vi "main mapping.vi"(8 "error in":errorcluster) -> (0 "error out":errorcluster)   [LabVIEW 2023]
uses:
  control/Data Form.ctl
  control/rois list cluster.ctl
  control/param_calibrazione.ctl
  <vilib>/Utility/miscctls.llb/LVStringsAndValuesArrayTypeDef_I16.ctl
  <vilib>/Utility/file.llb/Write Delimited Spreadsheet (I64).vi
  <vilib>/Utility/file.llb/Read Delimited Spreadsheet (string).vi
  queue/Front Panel Message Queue.lvlib
panel:
  in  "crop Z":bool
  in  "Crop Z sl":cluster{i32, i32}(slide) scale=0.0..10.0
  out "Invert Roi XY":bool[](array[boolean])
  out "Roi XY":T1
  in  "crop all":bool
  in  "crop":bool
  in  "save all":bool
  in  "save":bool
  in  "export":bool
  in  "Edit ROI":bool
  in  "autoscale":bool
  out "Calibration":T2
  in  "manipulate files":bool
  in  "area ROI":bool
  out "ROIs Values":string[][](table)
  out "data ROIs":T3
  out "ROIs Values Data":dbl[][](array[numeric])
  in  "ROIs List":i16(ring) items=["All", "Ca - Escape Peak", "S - Ka1", "Cl - Ka1", "Ar - Ka1", "K - Ka1", "Ca - Ka1", "Ca - Kb1", "Ti - Ka1", "Mn - Ka1", "Fe - Ka1", "Fe - Kb1", "Cu - Ka1", "Zn - Ka1"]
  in  "debug?":bool
  in  "load param":bool
  in  "load calib":bool
  in  "calibrate":bool
  in  "mapping":enum16{"Y - Linear", "Y - Log"}(ring)
  out "Intensity Graph":i32[][](graph)
  in  "reset":bool
  in  "reset ROI":bool
  out "Sum Spectrum":cluster{"Ramp Pattern":dbl[], "Array":i32[]}[](graph)
  in  "load data":bool
  in  "Data Form":T4={"Dimensions"={"Dim X"=0, "Dim Y"=0, "Dim Z"=0}, "Folder XRF Files"=path "", "Dynamic Load"=FALSE, "Data From Vitruvio?"=TRUE}
  in  "Z Slice":i16(slide) scale=0.0..10.0
  in  "Stop":bool
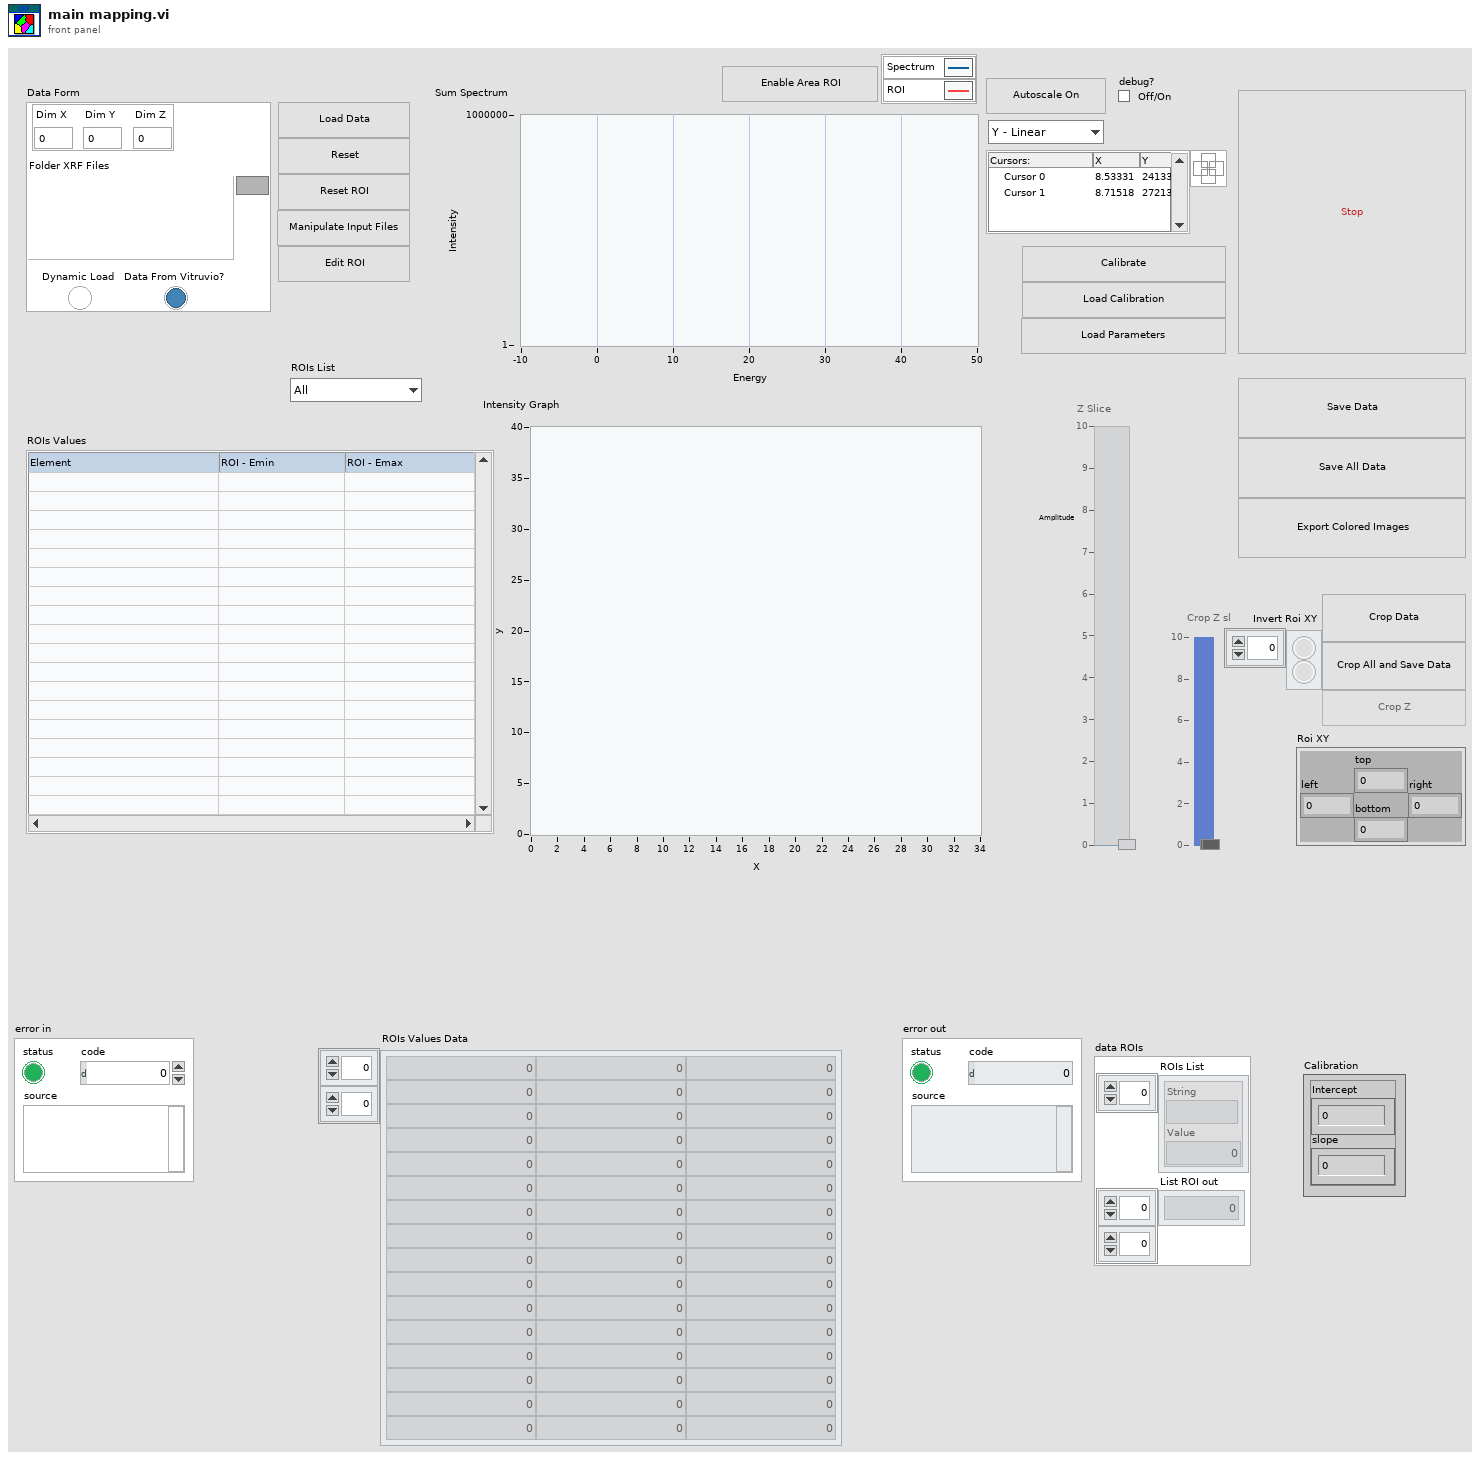
[diagram p1: front panel]
types:
  T1 = cluster{"left":i16, "top":i16, "right":i16, "bottom":i16}
  T2 = typedef "param_calibrazione.ctl" = cluster{"Intercept":dbl, "slope":dbl}
  T3 = typedef "rois list cluster.ctl" = cluster{"ROIs List":cluster{"String":string, "Value":i32}[], "List ROI out":dbl[][]}
  T4 = typedef "Data Form.ctl" = cluster{"Dimensions":cluster{"Dim X":i32, "Dim Y":i32, "Dim Z":i32}, "Folder XRF Files":path, "Dynamic Load":bool, "Data From Vitruvio?":bool}
  T5 = enum8{"Enabled", "Disabled", "Disabled and Grayed Out"}
  T6 = typedef "Front Panel Message Queue.lvlib/load 3 Messages Queues.ctl" = cluster{"Main":refnum<queue>, "Data":refnum<queue>, "Support":refnum<queue>}
  T7 = typedef "LVStringsAndValuesArrayTypeDef_I16.ctl" = cluster{"String":string, "Value":i16}[]
  T8 = typedef "LVRowAndColumnTypeDef.ctl" = cluster{"Row":i32, "Column":i32}
  T9 = typedef "LVCursorListTypeDef.ctl" = cluster{"Name":string, "Color":u32, "Style":u8, "Point Style":u8, "Name Visible":bool, "Allow Drag":bool, "Cursor Mode":u32, "Plot":i32, "Index":i32, "Position":cluster{"X":dbl, "Y":dbl}, "X Scale":u32, "Y Scale":u32, "Watch Plots":i32[], "Watch All Plots":bool, "Plot Area":i32, "Label Offset":cluster{"X":dbl, "Y":dbl}}[]
  T10 = cluster{"Name":string, "Color":u32, "Style":u8, "Point Style":u8, "Name Visible":bool, "Allow Drag":bool, "Cursor Mode":u32, "Plot":i32, "Index":i32, "Position":cluster{"X":dbl, "Y":dbl}, "X Scale":u32, "Y Scale":u32, "Watch Plots":i32[], "Watch All Plots":bool, "Plot Area":i32, "Label Offset":cluster{"X":dbl, "Y":dbl}}
  T11 = cluster{"Name":string, "Color":u32, "Style":u8, "Point Style":u8, "Name Visible":bool, "Allow Drag":bool, "Cursor Mode":u32, "Plot":i32, "Index":i32, "Position":cluster{"X":dbl, "Y":dbl}, "X Scale":u32, "Y Scale":u32, "Watch Plots":i32[], "Watch All Plots":bool, "Plot Area":i32, "Label Offset":cluster{"X":dbl, "Y":dbl}}[]
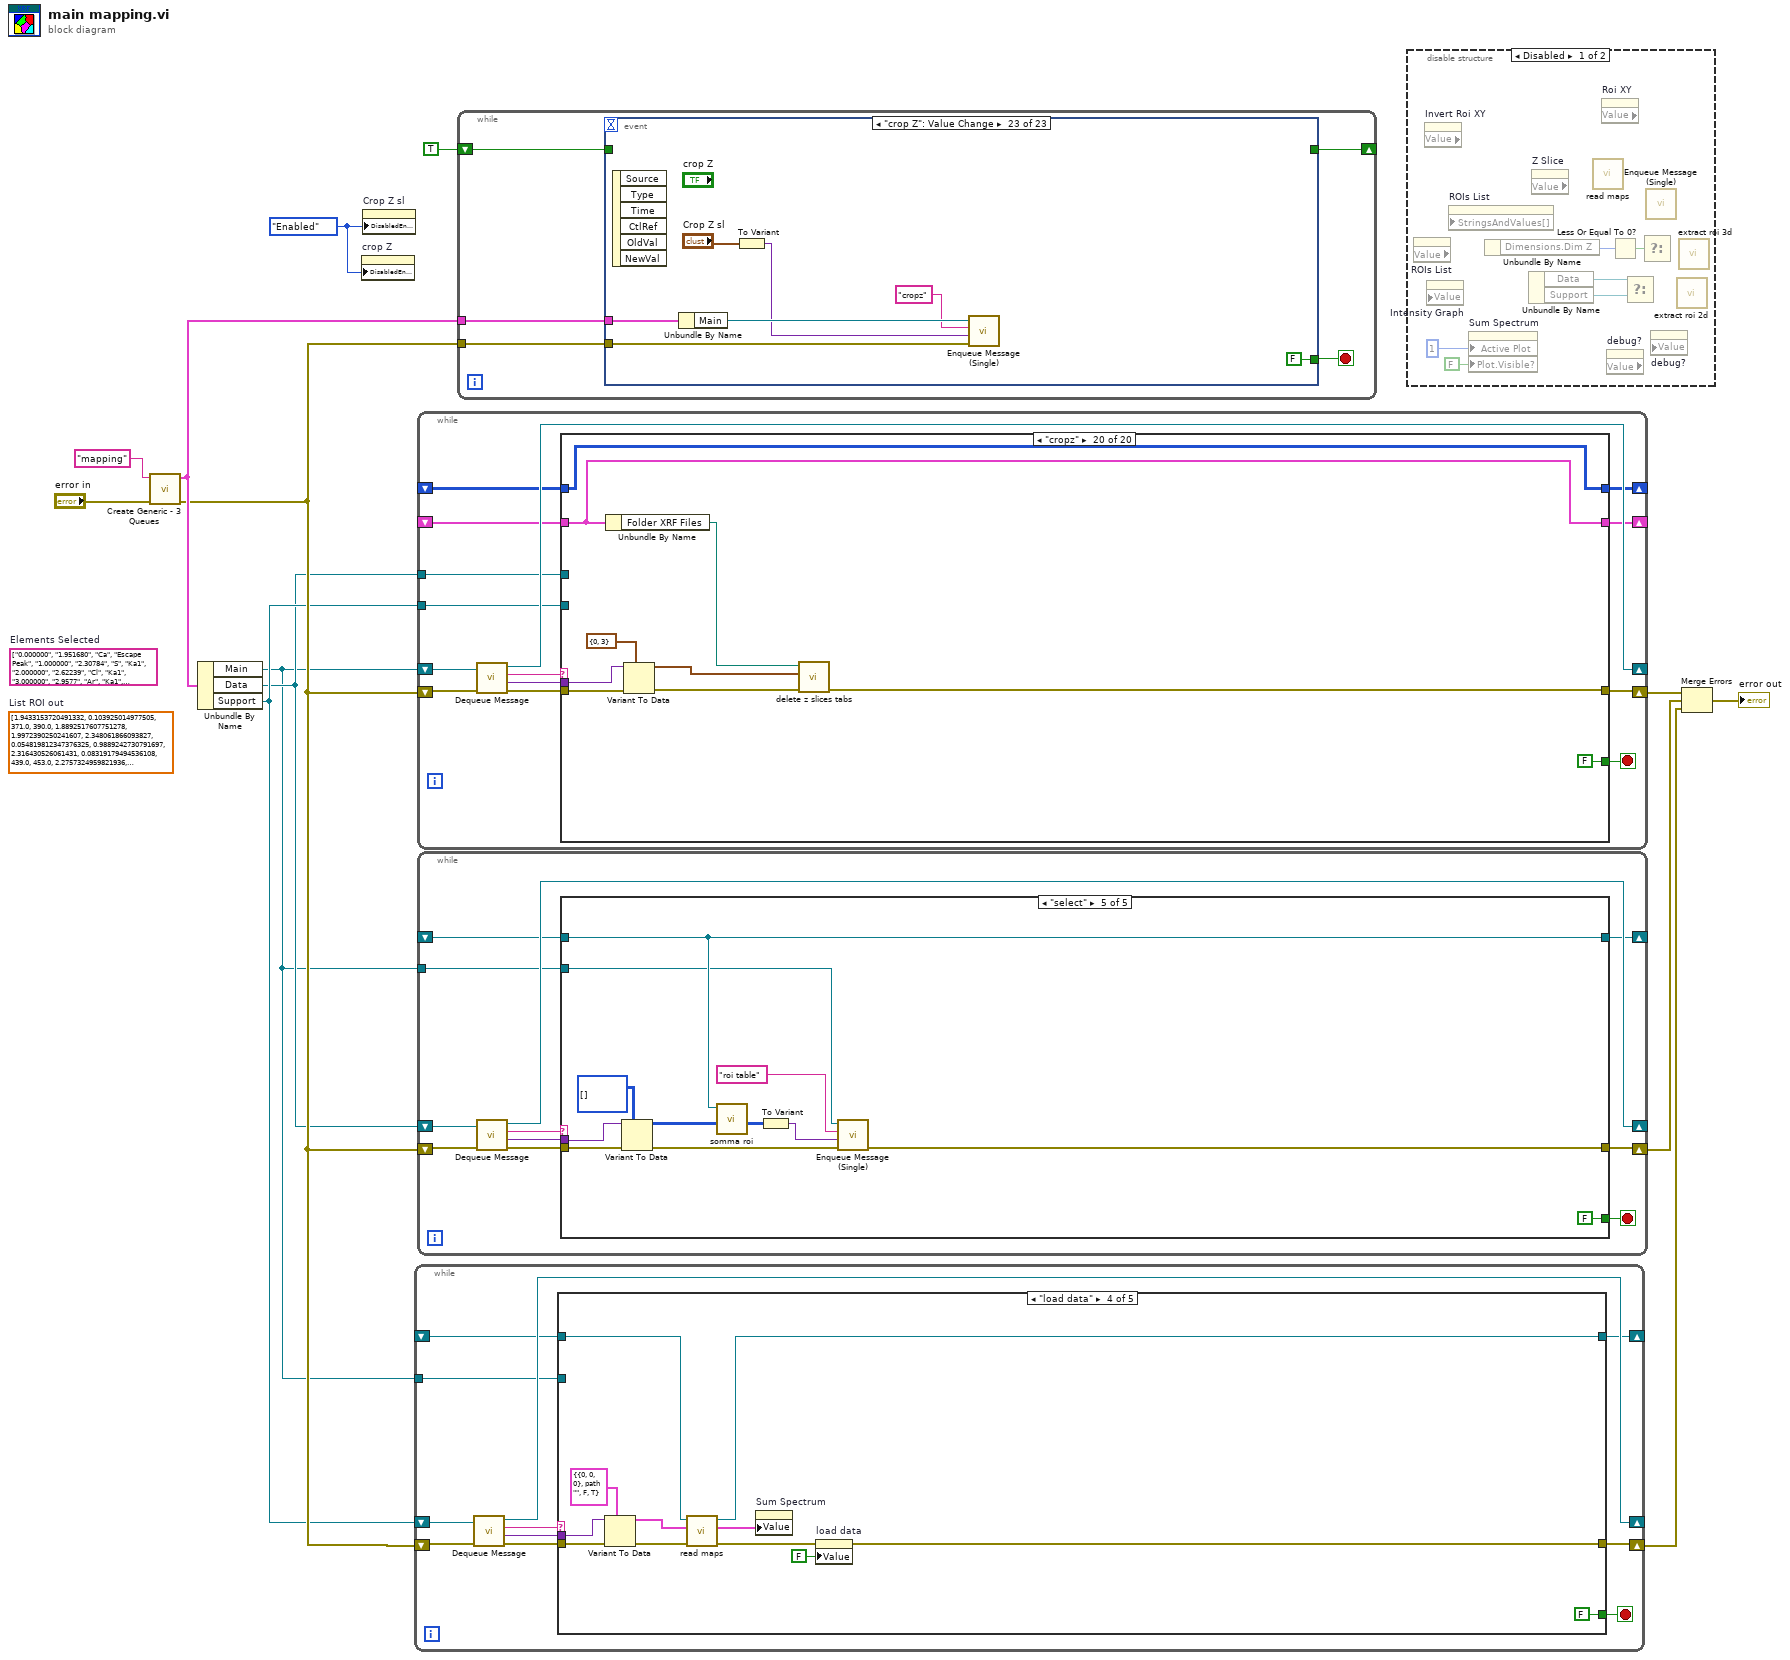
[diagram p0: block diagram]
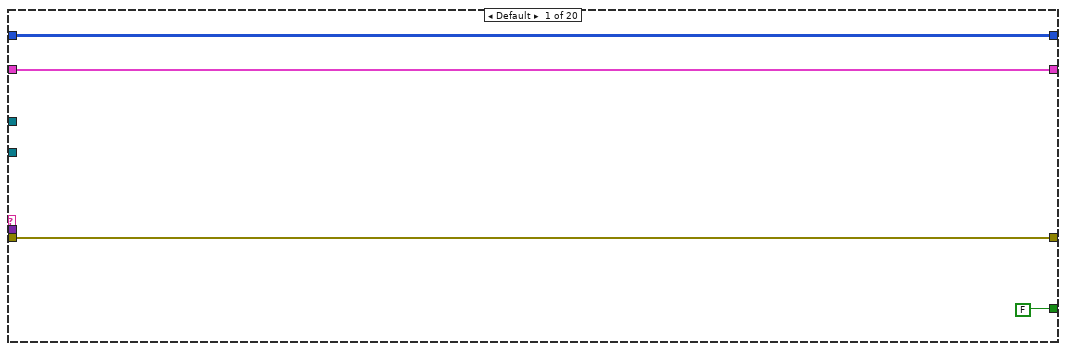
[diagram p3: hidden frame]
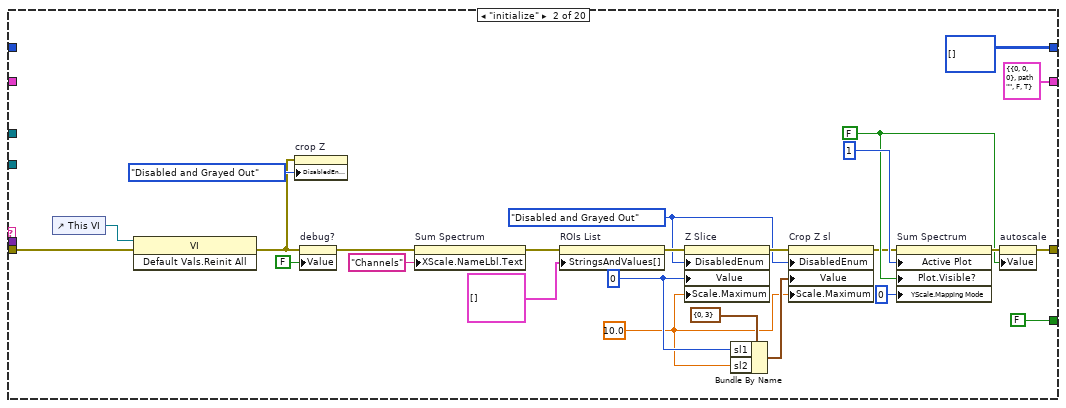
[diagram p4: hidden frame]
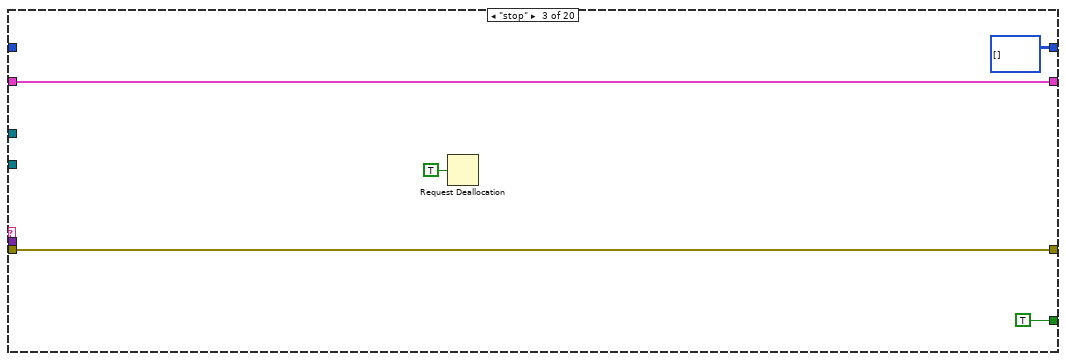
[diagram p5: hidden frame]
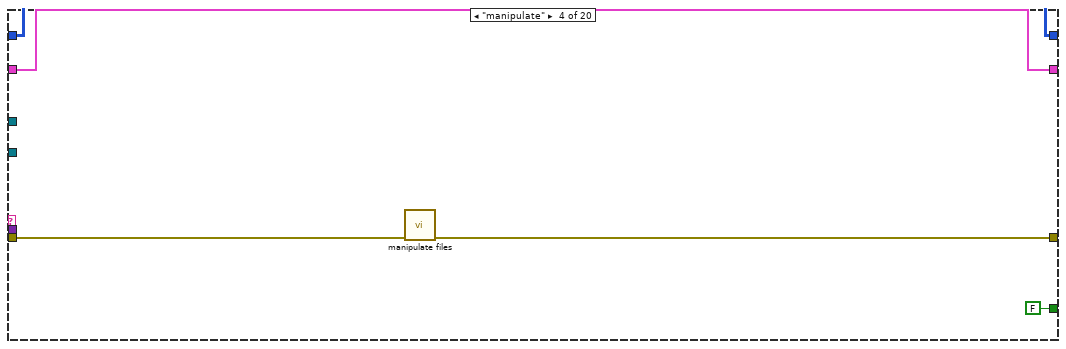
[diagram p6: hidden frame]
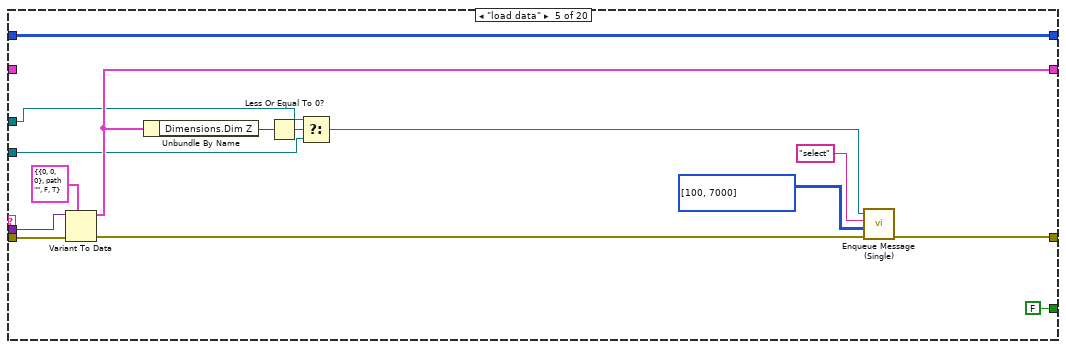
[diagram p7: hidden frame]
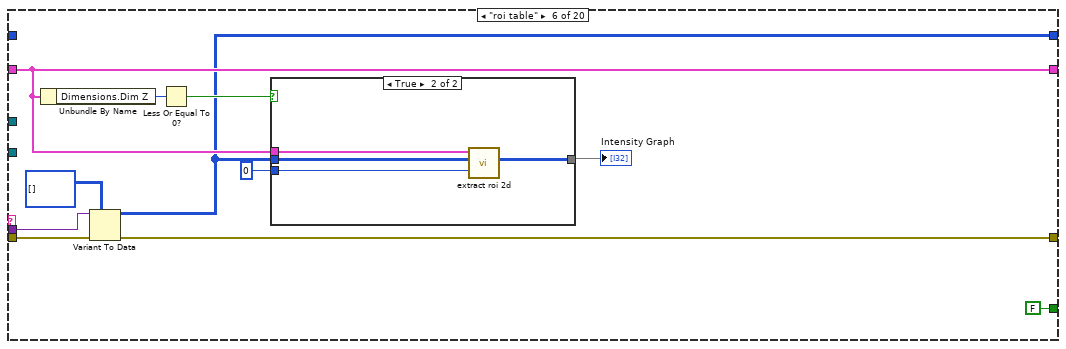
[diagram p8: hidden frame]
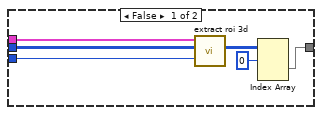
[diagram p9: hidden frame]
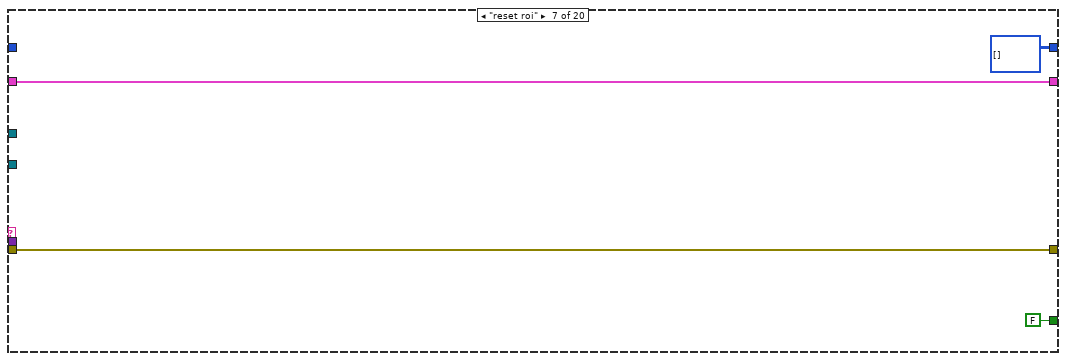
[diagram p10: hidden frame]
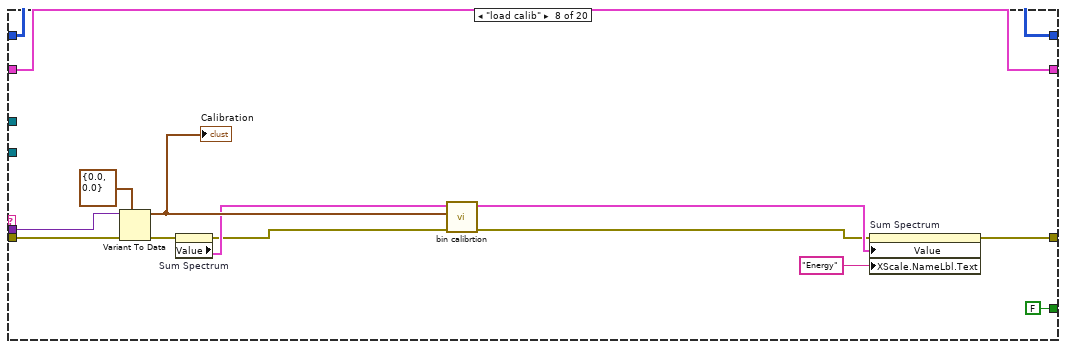
[diagram p11: hidden frame]
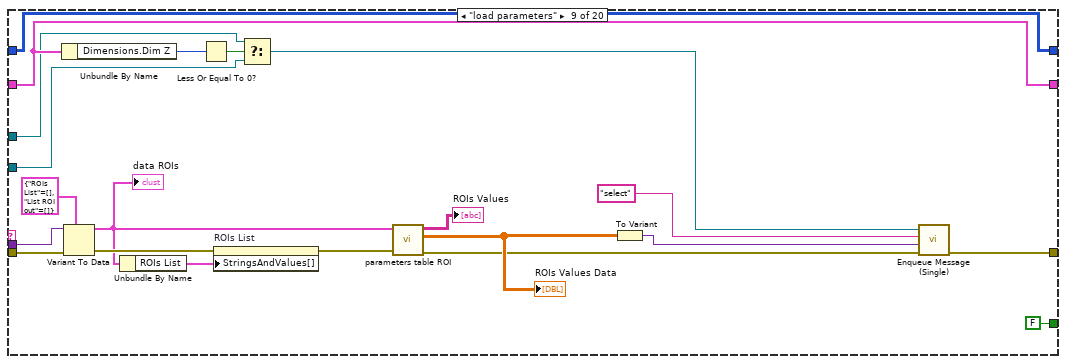
[diagram p12: hidden frame]
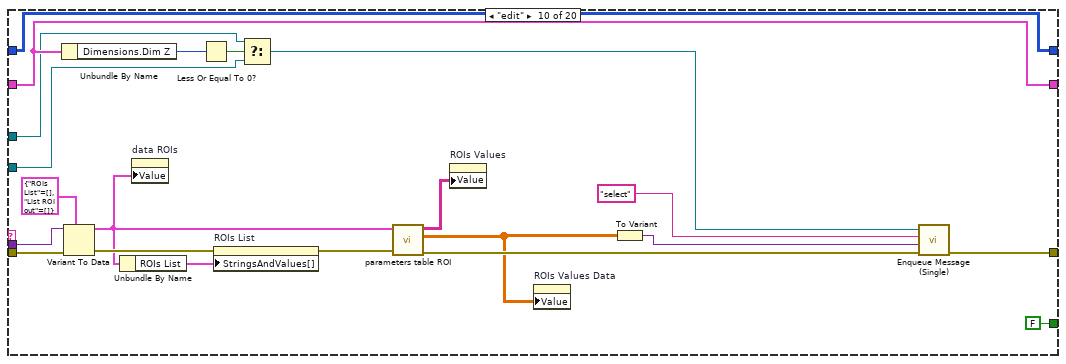
[diagram p13: hidden frame]
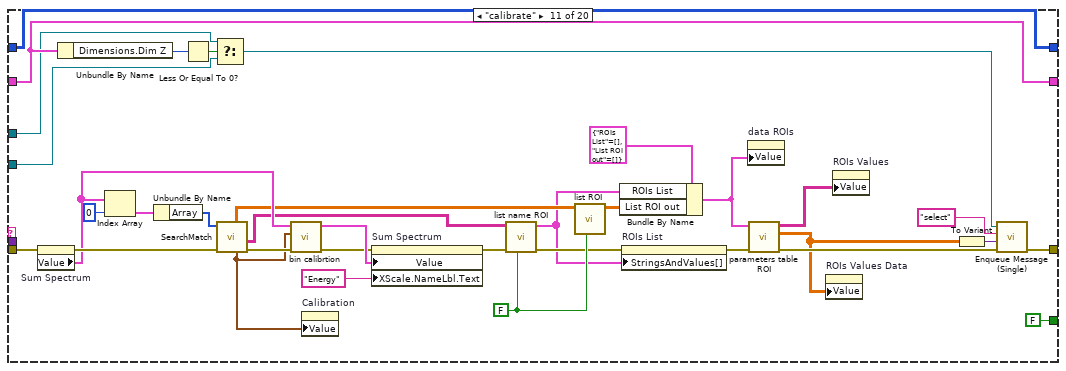
[diagram p14: hidden frame]
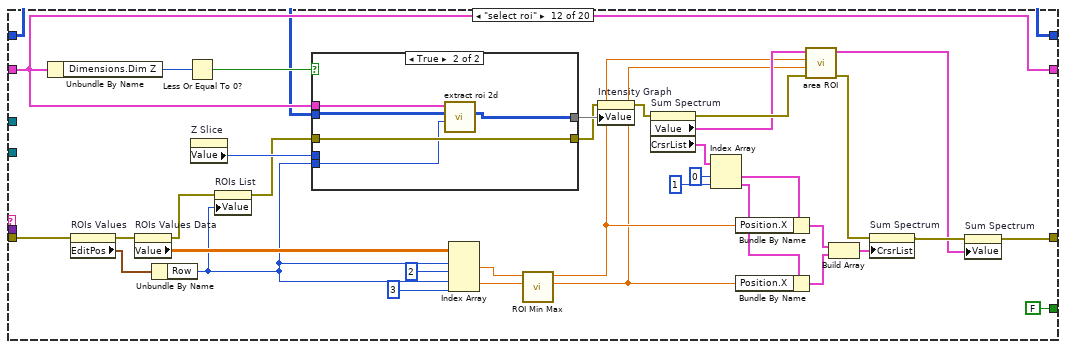
[diagram p15: hidden frame]
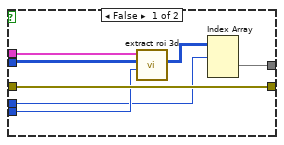
[diagram p16: hidden frame]
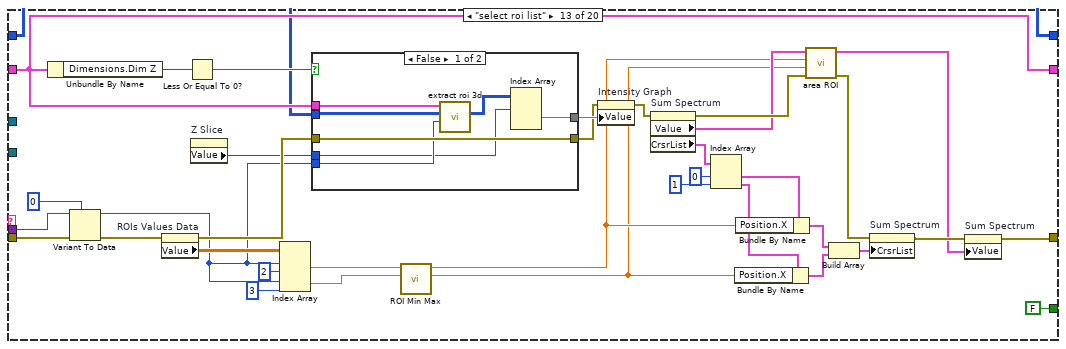
[diagram p17: hidden frame]
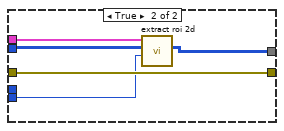
[diagram p18: hidden frame]
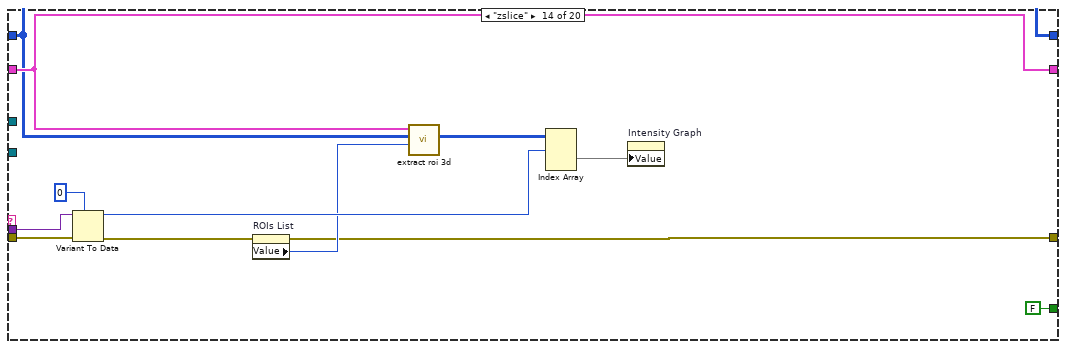
[diagram p19: hidden frame]
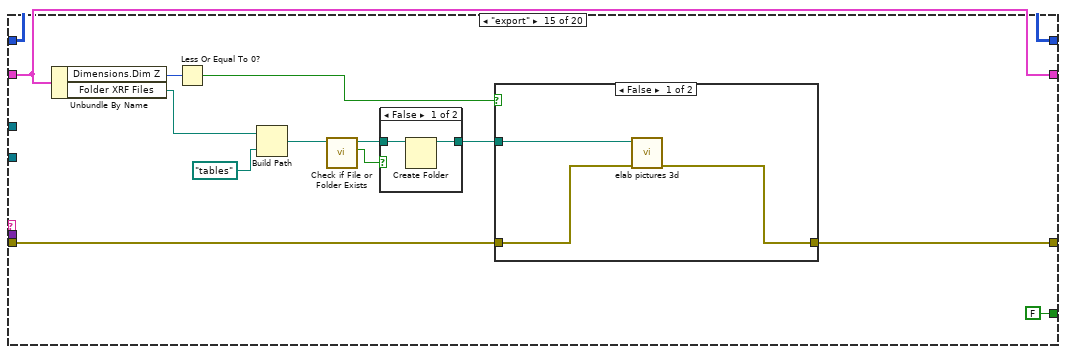
[diagram p20: hidden frame]
diagram:
  w1 = T5."Enabled" ("Disabled")
  (unwired) string[][] [["0.000000", "1.951680", "Ca", "Escape Peak"], ["1.000000", "2.30784", "S", "Ka1"], ["2.000000", "2.62239", "Cl", "Ka1"], ["3.000000", "2.9577", "Ar", "Ka1"], ["4.000000", "3.3138", "K", "Ka1"], ["5.000000", "3.69168", "Ca", "Ka1"], ["6.000000", "4.0127", "Ca", "Kb1"], ["7.000000", "4.51084", "Ti", "Ka1"], ["8.000000", "5.89875", "Mn", "Ka1"], ["9.000000", "6.40384", "Fe", "Ka1"], ["10.000000", "7.05798", "Fe", "Kb1"], ["11.000000", "8.04778", "Cu", "Ka1"], ["12.000000", "8.63886", "Zn", "Ka1"]]  # Elements Selected
  (unwired) dbl[][] [[1.9433153720491332, 0.103925014977505, 371.0, 390.0, 1.8892517607751278, 1.9972390250241607, 2.348061866093827, 0.054819812347376325, 0.9889242730791697], [2.316430526061431, 0.08319179494536108, 439.0, 453.0, 2.2757324959821936, 2.3553020591130602, 1.2026044683685715, 0.06508434345467039, 0.9422897397723133], [2.6291250873578926, 0.09464714383641912, 493.0, 510.0, 2.5826436680583935, 2.67926385186016, 6.041240478814808, 0.09369315412168325, 0.9948773271231875], [2.9638857471497273, 0.10205305258568396, 551.0, 569.0, 2.912289001029126, 3.0145927250545257, 19.912809301577955, 0.16530990532407933, 0.9985039668315457], [3.315602816840393, 0.10433962779562063, 613.0, 631.0, 3.264668494894392, 3.366972218919792, 7.760413909880946, 0.3328586753679668, 0.960961680843631], [3.695302221205313, 0.11473980336266298, 679.0, 699.0, 3.6397821496541916, 3.7534529541268578, 209.52164584521063, 0.9542698579126939, 0.9995310820008576], [4.016866195819118, 0.11712275853598021, 735.0, 756.0, 3.9580604021776575, 4.0774147468739566, 31.75496431275371, 0.47134819167031033, 0.9949696927449659], [4.512431596555036, 0.12331628047684387, 822.0, 843.0, 4.4525284016337565, 4.571882746330056, 2.030401395630214, 0.06554154967612931, 0.9764849440574406], [5.899492088990847, 0.14789502732767537, 1064.0, 1090.0, 5.827945135753021, 5.975717181567487, 2.129686188635054, 0.14744421626074894, 0.8984068833785415], [6.3992920200960155, 0.14207300042877877, 1152.0, 1177.0, 6.328096675432753, 6.470185181023586, 53.24985306608518, 0.5108773919278868, 0.9977288374603356], [7.060693940644275, 0.1502701906643122, 1268.0, 1294.0, 6.987387341374219, 7.135159387188685, 7.411818206694545, 0.3851918524072267, 0.9365265800601416], [8.037279832035043, 0.15266067897053234, 1439.0, 1466.0, 7.959272719615518, 8.112728305653617, 8.778131477093314, 0.519491476790709, 0.9143052423937907], [8.624129113105631, 0.1800441786593039, 1540.0, 1572.0, 8.533310282202482, 8.715183569358748, 10.127705234792012, 0.49635854961799064, 0.9435596103561451]]  # List ROI out
  n1 = call "Create Generic - 3 Queues.vi"("error in (no error)"="error in", "name"="mapping") -> ("error out"=w7:errorcluster, "Message Queues"=w11:T6)  [unwired: 8 in]
  n2 = Unbundle By Name(w11) -> ("Main"=w2:refnum<queue>, "Data"=w5:refnum<queue>, "Support"=w6:refnum<queue>)
  n3 = property on="crop Z" class="Bool"("DisabledEnum"=w1) -> ()  [unwired: 2 in, 2 out]
  n4 = property on="Crop Z sl" class="Slide (strict)"("DisabledEnum"=w1) -> ()  [unwired: 2 in, 2 out]
  n5 = while {
    shift-right: [w22] -> _
    shift-left: w6 -> [w23]
    shift-right: [w17] -> w9
    shift-left: w7 -> [w24]
    shift-right: [w16] -> _
    shift-left: _ -> [w15]
    tunnel: w2 -> [w14]
    stop <- w19 stop-if-true
    n6 = call "Dequeue Message.vi"("error in (no error)"=w24, "Message Queue"=w23) -> ("error out"=w21:errorcluster, "Message Data"=w18:variant, "Message"=w20:string, "dup Message Queue"=w22:refnum<queue>)  [unwired: 5 in, 1 out]
    n7 = case shown="\"load data\"" w20 {
      tunnel: w21 -> [w26 w28 w36 w47 w58]
      tunnel: [FALSE FALSE TRUE FALSE FALSE] -> w19
      tunnel: w18 -> [_ _ _ w46 w59]
      tunnel: [w26 w29 w35 w38 w50] -> w17
      tunnel: [w25 w30 refnum<data-value> refnum ("data value reference out") w41 w57] -> w16
      tunnel: w15 -> [w25 _ w34 w44 w57]
      tunnel: w14 -> [_ _ _ _ w51]
      frame Default {
      }
      frame "initialize" {
        n8 = New Data Value Reference(data value=i32[][] [] ("Data Loaded"), error in=w28) -> (data value reference=w30:refnum<data-value>, error out=w29:errorcluster)
      }
      frame "stop" {
        n9 = Delete Data Value Reference(data value reference=w34, error in=w36) -> (error out=w35:errorcluster)  [unwired: 1 out]
      }
      frame "load data" {
        n10 = Variant To Data(error in=w47, type=T4 {"Dimensions"={"Dim X"=0, "Dim Y"=0, "Dim Z"=0}, "Folder XRF Files"=path "", "Dynamic Load"=FALSE, "Data From Vitruvio?"=TRUE} ("Data Form"), Variant=w46) -> (data=w43:T4, error out=w45:errorcluster)
        n11 = call "read maps.vi"("error in"=w45, "Data Form"=w43, "data value reference In"=w44) -> ("error out"=w39:errorcluster, "All Spectra"=w42:cluster{"Ramp Pattern":dbl[], "Array":i32[]}[], "data value reference out"=w41:refnum<data-value>)  [unwired: 6 in]
        n12 = property on="Sum Spectrum" class="XYGraph (strict)"("Value"=w42) -> ()  [unwired: 2 in, 2 out]
        n13 = property on="load data" class="Bool (strict)"(error in=w39, "Value"=FALSE ("load data")) -> (error out=w38:errorcluster)  [unwired: 1 in, 1 out]
      }
      frame "select" {
        n14 = Variant To Data(error in=w58, type=i32[][] [] ("ROIs Min Max"), Variant=w59) -> (data=w56:i32[][], error out=w53:errorcluster)
        n15 = call "somma roi.vi"("ROIs Min Max"=w56, "Data loaded reference In"=w57) -> ("ROIs Array Out"=w52:i32[][])  [unwired: 9 in]
        n16 = To Variant(anything=w52) -> (Variant=w55:variant)
        n17 = call "Enqueue Message (Single).vi"("error in (no error)"=w53, "Message Data"=w55, "Message"="roi table", "Message Queue"=w51) -> ("error out"=w50:errorcluster)  [unwired: 6 in, 1 out]
      }
    }
  }
  n18 = while {
    shift-right: [w73] -> _
    shift-left: w2 -> [w74]
    shift-right: [w68] -> w4
    shift-left: w7 -> [w75]
    tunnel: w6 -> [w66]
    tunnel: w5 -> [w67]
    shift-right: [w65] -> _
    shift-left: _ -> [w64]
    shift-right: [w63] -> _
    shift-left: _ -> [w62]
    stop <- w70 stop-if-true
    n19 = call "Dequeue Message.vi"("error in (no error)"=w75, "Message Queue"=w74) -> ("error out"=w72:errorcluster, "Message Data"=w69:variant, "Message"=w71:string, "dup Message Queue"=w73:refnum<queue>)  [unwired: 5 in, 1 out]
    n20 = case shown="\"cropz\"" w71 {
      tunnel: w72 -> [w78 w100 w109 w113 w128 w138 w153 w163 w182 w203 w238 w280 w300 w350 w362 w391 w436 w490 w520 w583]
      tunnel: [FALSE FALSE TRUE FALSE FALSE FALSE FALSE FALSE FALSE FALSE FALSE FALSE FALSE FALSE FALSE FALSE FALSE FALSE FALSE FALSE] -> w70
      tunnel: w69 -> [_ _ _ _ w127 w137 _ w161 w180 w201 _ _ w301 w349 _ _ _ _ _ w581]
      tunnel: [w78 w91 w109 w112 w119 w130 w153 w166 w176 w197 w221 w261 w311 w342 w361 w390 w435 w485 w521 w575] -> w68
      tunnel: w67 -> [_ _ _ _ w121 _ _ _ w184 w205 w240 _ _ _ _ _ _ _ _ _]
      tunnel: w66 -> [_ _ _ _ w120 _ _ _ w183 w204 w239 _ _ _ _ _ _ _ _ _]
      tunnel: [w77 T4 {"Dimensions"={"Dim X"=0, "Dim Y"=0, "Dim Z"=0}, "Folder XRF Files"=path "", "Dynamic Load"=FALSE, "Data From Vitruvio?"=TRUE} ("Data Form") w106 w110 w122 w134 w152 w164 w186 w207 w241 w272 w323 w352 w363 w382 w427 w494 w523 w577] -> w65
      tunnel: w64 -> [w77 _ w106 w110 _ w134 w152 w164 w186 w207 w241 w272 w323 w352 w363 w382 w427 w494 w523 w577]
      tunnel: [w76 i32[][] [] ("ROIs Array Out") i32[][] [] ("ROIs Array Out") w111 w125 w131 i32[][] [] ("ROIs Array Out") w165 w188 w209 w244 w270 w320 w351 w365 w381 w426 w493 w522 w578] -> w63
      tunnel: w62 -> [w76 _ _ w111 w125 _ _ w165 w188 w209 w244 w270 w320 w351 w365 w381 w426 w493 w522 w578]
      frame Default {
      }
      frame "initialize" {
        w82 = 10.0 ("Scale.Range:Maximum")
        w84 = i16 0 ("Z Slice")
        w90 = FALSE ("Plot.Visible")
        w86 = T5."Disabled and Grayed Out" ("Disabled")
        n21 = control-ref of="This VI"() -> (w99:refnum<vi>)
        n22 = invoke class="VI" method="Default Vals.Reinit All"(reference=w99, error in=w100) -> (error out=w80:errorcluster)  [unwired: 1 in, 2 out]
        n23 = property on="crop Z" class="Bool"(error in=w80, "DisabledEnum"=T5."Disabled and Grayed Out" ("Disabled")) -> ()  [unwired: 1 in, 2 out]
        n24 = property on="debug?" class="Bool (strict)"(error in=w80, "Value"=FALSE ("debug?")) -> (error out=w98:errorcluster)  [unwired: 1 in, 1 out]
        n25 = property on="Sum Spectrum" class="XYGraph (strict)"(error in=w98, "XScale.NameLbl.Text"="Channels" ("X Scale.Name Label.Text")) -> (error out=w96:errorcluster)  [unwired: 1 in, 1 out]
        n26 = property on="ROIs List" class="Ring (strict)"(error in=w96, "StringsAndValues[]"=T7 [] ("Strings And Values []")) -> (error out=w94:errorcluster)  [unwired: 1 in, 1 out]
        n27 = property on="Z Slice" class="Slide (strict)"(error in=w94, "DisabledEnum"=w86, "Value"=w84, "Scale.Maximum"=w82) -> (error out=w87:errorcluster)  [unwired: 1 in, 1 out]
        n28 = Bundle By Name(cluster=cluster{"sl1":i32, "sl2":i32} {"sl1"=0, "sl2"=3} ("Crop Z"), "sl1"=w84, "sl2"=w82) -> (w83:cluster{"sl1":i32, "sl2":i32})
        n29 = property on="Crop Z sl" class="Slide (strict)"(error in=w87, "DisabledEnum"=w86, "Value"=w83, "Scale.Maximum"=w82) -> (error out=w88:errorcluster)  [unwired: 1 in, 1 out]
        n30 = property on="Sum Spectrum" class="XYGraph (strict)"(error in=w88, "Active Plot"=u32 1, "Plot.Visible?"=w90, "YScale.Mapping Mode"=u8 0 ("Y Scale.Mapping Mode")) -> (error out=w92:errorcluster)  [unwired: 1 in, 1 out]
        n31 = property on="autoscale" class="Bool (strict)"(error in=w92, "Value"=w90) -> (error out=w91:errorcluster)  [unwired: 1 in, 1 out]
      }
      frame "stop" {
        n32 = Request Deallocation(TRUE ("flag")) -> ()
      }
      frame "manipulate" {
        n33 = call "manipulate files.vi"("error in"=w113) -> ("error out"=w112:errorcluster)  [unwired: 10 in]
      }
      frame "load data" {
        n34 = Variant To Data(error in=w128, type=T4 {"Dimensions"={"Dim X"=0, "Dim Y"=0, "Dim Z"=0}, "Folder XRF Files"=path "", "Dynamic Load"=FALSE, "Data From Vitruvio?"=TRUE} ("Data Form"), Variant=w127) -> (data=w122:T4, error out=w118:errorcluster)
        n35 = Unbundle By Name(w122) -> ("Dimensions.Dim Z"=w124:i32)
        n36 = Less Or Equal To 0?(x=w124) -> (x <= 0?=w123:bool)
        n37 = Select(t=w121, s=w123, f=w120) -> (s? t:f=w117:refnum<queue>)
        n38 = call "Enqueue Message (Single).vi"("error in (no error)"=w118, "Message Data"=i32[][] [[100, 7000]] ("ROIs Min Max"), "Message"="select", "Message Queue"=w117) -> ("error out"=w119:errorcluster)  [unwired: 6 in, 1 out]
      }
      frame "roi table" {
        n39 = Unbundle By Name(w134) -> ("Dimensions.Dim Z"=w139:i32)
        n40 = Variant To Data(error in=w138, type=i32[][] [] ("ROIs Array Out"), Variant=w137) -> (data=w131:i32[][], error out=w130:errorcluster)
        n41 = Less Or Equal To 0?(x=w139) -> (x <= 0?=w135:bool)
        n42 = case shown="True" w135 {
          tunnel: w134 -> [w146 w150]
          tunnel: [w143 w149] -> w133
          tunnel: w131 -> [w142 w148]
          tunnel: i16 0 -> [w141 w147]
          frame False {
            n43 = call "extract roi 3d.vi"("ROI selected"=w141, "ROIs Array In"=w142, "Data Form"=w146) -> ("Table ROI 3D"=w145:i32[][][])  [unwired: 8 in]
            n44 = Index Array(array=w145, index (dim 0)=0 ("index (page)")) -> (element=w143:i32[][])  [unwired: 2 in]
          }
          frame True {
            n45 = call "extract roi 2d.vi"("ROI selected"=w147, "ROIs Array In"=w148, "Data Form"=w150) -> ("Table ROI 2D"=w149:i32[][])  [unwired: 8 in]
          }
        }
        "Intensity Graph" <- w133
      }
      frame "reset roi" {
      }
      frame "load calib" {
        n46 = Variant To Data(error in=w163, type=T2 {"Intercept"=0.0, "slope"=0.0} ("Param Calibrazione"), Variant=w161) -> (data=w159:T2, error out=w162:errorcluster)
        "Calibration" <- w159
        n47 = property on="Sum Spectrum" class="XYGraph (strict)"(error in=w162) -> (error out=w156:errorcluster, "Value"=w158:cluster{"Ramp Pattern":dbl[], "Array":i32[]}[])  [unwired: 1 in, 1 out]
        n48 = call "bin calibrtion.vi"("error in"=w156, "Param Calibrazione"=w159, "Sum Spectrum"=w158) -> ("error out"=w155:errorcluster, "Sum Spectrum Out"=w157:cluster{"Ramp Pattern":dbl[], "Array":i32[]}[])  [unwired: 7 in]
        n49 = property on="Sum Spectrum" class="XYGraph (strict)"(error in=w155, "Value"=w157, "XScale.NameLbl.Text"="Energy" ("X Scale.Name Label.Text")) -> (error out=w166:errorcluster)  [unwired: 1 in, 1 out]
      }
      frame "load parameters" {
        n50 = Unbundle By Name(w186) -> ("Dimensions.Dim Z"=w187:i32)
        n51 = Variant To Data(error in=w182, type=T3 {"ROIs List"=[], "List ROI out"=[]}, Variant=w180) -> (data=w170:T3, error out=w171:errorcluster)
        "data ROIs" <- w170
        n52 = Unbundle By Name(w170) -> ("ROIs List"=w169:cluster{"String":string, "Value":i32}[])
        n53 = Less Or Equal To 0?(x=w187) -> (x <= 0?=w185:bool)
        n54 = property on="ROIs List" class="Ring (strict)"(error in=w171, "StringsAndValues[]"=w169) -> (error out=w172:errorcluster)  [unwired: 1 in, 1 out]
        n55 = Select(t=w184, s=w185, f=w183) -> (s? t:f=w178:refnum<queue>)
        n56 = call "parameters table ROI.vi"("error in"=w172, "data ROIs"=w170) -> ("error out"=w174:errorcluster, "ROIs Values Data"=w175:dbl[][], "ROIs Values"=→"ROIs Values":string[][])  [unwired: 7 in]
        "ROIs Values Data" <- w175
        n57 = To Variant(anything=w175) -> (Variant=w179:variant)
        n58 = call "Enqueue Message (Single).vi"("error in (no error)"=w174, "Message Data"=w179, "Message"="select", "Message Queue"=w178) -> ("error out"=w176:errorcluster)  [unwired: 6 in, 1 out]
      }
      frame "edit" {
        n59 = Unbundle By Name(w207) -> ("Dimensions.Dim Z"=w208:i32)
        n60 = Variant To Data(error in=w203, type=T3 {"ROIs List"=[], "List ROI out"=[]}, Variant=w201) -> (data=w192:T3, error out=w194:errorcluster)
        n61 = Unbundle By Name(w192) -> ("ROIs List"=w193:cluster{"String":string, "Value":i32}[])
        n62 = property on="data ROIs" class="Clust (strict)"("Value"=w192) -> ()  [unwired: 2 in, 2 out]
        n63 = Less Or Equal To 0?(x=w208) -> (x <= 0?=w206:bool)
        n64 = property on="ROIs List" class="Ring (strict)"(error in=w194, "StringsAndValues[]"=w193) -> (error out=w195:errorcluster)  [unwired: 1 in, 1 out]
        n65 = Select(t=w205, s=w206, f=w204) -> (s? t:f=w199:refnum<queue>)
        n66 = call "parameters table ROI.vi"("error in"=w195, "data ROIs"=w192) -> ("error out"=w196:errorcluster, "ROIs Values Data"=w190:dbl[][], "ROIs Values"=w191:string[][])  [unwired: 7 in]
        n67 = property on="ROIs Values" class="Tbl (strict)"("Value"=w191) -> ()  [unwired: 2 in, 2 out]
        n68 = property on="ROIs Values Data" class="Arr (strict)"("Value"=w190) -> ()  [unwired: 2 in, 2 out]
        n69 = To Variant(anything=w190) -> (Variant=w200:variant)
        n70 = call "Enqueue Message (Single).vi"("error in (no error)"=w196, "Message Data"=w200, "Message"="select", "Message Queue"=w199) -> ("error out"=w197:errorcluster)  [unwired: 6 in, 1 out]
      }
      frame "calibrate" {
        w223 = FALSE ("debug?")
        n71 = property on="Sum Spectrum" class="XYGraph (strict)"(error in=w238) -> (error out=w237:errorcluster, "Value"=w229:cluster{"Ramp Pattern":dbl[], "Array":i32[]}[])  [unwired: 1 in, 1 out]
        n72 = Unbundle By Name(w241) -> ("Dimensions.Dim Z"=w243:i32)
        n73 = Index Array(array=w229, index=0) -> (element=w235:cluster{"Ramp Pattern":dbl[], "Array":i32[]})
        n74 = Unbundle By Name(w235) -> ("Array"=w234:i32[])
        n75 = Less Or Equal To 0?(x=w243) -> (x <= 0?=w242:bool)
        n76 = Select(t=w240, s=w242, f=w239) -> (s? t:f=w219:refnum<queue>)
        n77 = call "SearchMatch.vi"("Error In"=w237, "data_from2d3d"=w234) -> ("Error Out"=w230:errorcluster, "Elements Selected"=w227:string[][], "Param Calibrazione"=w213:T2, "List ROI out"=w226:dbl[][])  [unwired: 5 in, 1 out]
        n78 = call "bin calibrtion.vi"("error in"=w230, "Param Calibrazione"=w213, "Sum Spectrum"=w229) -> ("error out"=w232:errorcluster, "Sum Spectrum Out"=w233:cluster{"Ramp Pattern":dbl[], "Array":i32[]}[])  [unwired: 7 in]
        n79 = property on="Calibration" class="Clust (strict)"("Value"=w213) -> ()  [unwired: 2 in, 2 out]
        n80 = property on="Sum Spectrum" class="XYGraph (strict)"(error in=w232, "Value"=w233, "XScale.NameLbl.Text"="Energy" ("X Scale.Name Label.Text")) -> (error out=w228:errorcluster)  [unwired: 1 in, 1 out]
        n81 = call "list name ROI.vi"("debug?"=w223, "error in"=w228, "Elements Selected"=w227) -> ("error out"=w215:errorcluster, "ROIs List"=w212:cluster{"String":string, "Value":i32}[])  [unwired: 7 in]
        n82 = call "list ROI.vi"("debug?"=w223, "List ROI in"=w226) -> ("List ROI out"=w224:dbl[][])  [unwired: 9 in]
        n83 = Bundle By Name(cluster=T3 {"ROIs List"=[], "List ROI out"=[]}, "ROIs List"=w212, "List ROI out"=w224) -> (w211:T3)
        n84 = property on="ROIs List" class="Ring (strict)"(error in=w215, "StringsAndValues[]"=w212) -> (error out=w214:errorcluster)  [unwired: 1 in, 1 out]
        n85 = property on="data ROIs" class="Clust (strict)"("Value"=w211) -> ()  [unwired: 2 in, 2 out]
        n86 = call "parameters table ROI.vi"("error in"=w214, "data ROIs"=w211) -> ("error out"=w220:errorcluster, "ROIs Values Data"=w216:dbl[][], "ROIs Values"=w222:string[][])  [unwired: 7 in]
        n87 = property on="ROIs Values Data" class="Arr (strict)"("Value"=w216) -> ()  [unwired: 2 in, 2 out]
        n88 = property on="ROIs Values" class="Tbl (strict)"("Value"=w222) -> ()  [unwired: 2 in, 2 out]
        n89 = To Variant(anything=w216) -> (Variant=w217:variant)
        n90 = call "Enqueue Message (Single).vi"("error in (no error)"=w220, "Message Data"=w217, "Message"="select", "Message Queue"=w219) -> ("error out"=w221:errorcluster)  [unwired: 6 in, 1 out]
      }
      frame "select roi" {
        n91 = Unbundle By Name(w272) -> ("Dimensions.Dim Z"=w274:i32)
        n92 = property on="ROIs Values" class="Tbl (strict)"(error in=w280) -> (error out=w278:errorcluster, "EditPos"=w279:T8)  [unwired: 1 in, 1 out]
        n93 = property on="ROIs Values Data" class="Arr (strict)"(error in=w278) -> (error out=w248:errorcluster, "Value"=w277:dbl[][])  [unwired: 1 in, 1 out]
        n94 = Unbundle By Name(w279) -> ("Row"=w246:i32)
        n95 = Less Or Equal To 0?(x=w274) -> (x <= 0?=w273:bool)
        n96 = property on="Z Slice" class="Slide (strict)"() -> ("Value"=w271:i16)  [unwired: 2 in, 2 out]
        n97 = property on="ROIs List" class="Ring (strict)"(error in=w248, "Value"=w246) -> (error out=w247:errorcluster)  [unwired: 1 in, 1 out]
        n98 = case shown="True" w273 {
          tunnel: w270 -> [w288 w292]
          tunnel: w247 -> [w286 w291]
          tunnel: w272 -> [w287 w293]
          tunnel: [w286 w291] -> w268
          tunnel: [w284 w290] -> w269
          tunnel: w271 -> [w282 _]
          tunnel: w246 -> [w283 w289]
          frame False {
            n99 = call "extract roi 3d.vi"("ROI selected"=w283, "ROIs Array In"=w288, "Data Form"=w287) -> ("Table ROI 3D"=w285:i32[][][])  [unwired: 8 in]
            n100 = Index Array(array=w285, index (dim 0)=w282) -> (element=w284:i32[][])  [unwired: 2 in]
          }
          frame True {
            n101 = call "extract roi 2d.vi"("ROI selected"=w289, "ROIs Array In"=w292, "Data Form"=w293) -> ("Table ROI 2D"=w290:i32[][])  [unwired: 8 in]
          }
        }
        n102 = Index Array(array=w277, index (row) #1=w246, index (col) #1=2 ("disabled index (col)"), index (row) #2=w246, index (col) #2=3 ("index (col)")) -> (element #1=w252:dbl, element #2=w251:dbl)
        n103 = call "ROI Min Max.vi"("ROI 2"=w251, "ROI 1"=w252) -> ("ROI Max"=w249:dbl, "ROI Min"=w250:dbl)  [unwired: 8 in]
        n104 = property on="Intensity Graph" class="IntGraph (strict)"(error in=w268, "Value"=w269) -> (error out=w256:errorcluster)  [unwired: 1 in, 1 out]
        n105 = property on="Sum Spectrum" class="XYGraph (strict)"(error in=w256) -> (error out=w257:errorcluster, "Value"=w255:cluster{"Ramp Pattern":dbl[], "Array":i32[]}[], "CrsrList"=w253:T9)  [unwired: 1 in, 1 out]
        n106 = Index Array(array=w253, index #1=0 ("index"), index #2=1 ("index")) -> (element #1=w265:T10, element #2=w264:T10)
        n107 = Bundle By Name(cluster=w265, "Position.X"=w250) -> (w263:T10)
        n108 = Bundle By Name(cluster=w264, "Position.X"=w249) -> (w262:T10)
        n109 = call "area ROI.vi"("error in"=w257, "ROI max"=w249, "ROI min"=w250, "Sum Spectrum"=w255) -> ("error out"=w254:errorcluster, "XY Graph"=w259:cluster{"Channel":dbl[], "Intensity":i32[]}[])  [unwired: 5 in, 1 out]
        n110 = Build Array(w263, w262) -> (w258:T11)
        n111 = property on="Sum Spectrum" class="XYGraph (strict)"(error in=w254, "CrsrList"=w258) -> (error out=w260:errorcluster)  [unwired: 1 in, 1 out]
        n112 = property on="Sum Spectrum" class="XYGraph (strict)"(error in=w260, "Value"=w259) -> (error out=w261:errorcluster)  [unwired: 1 in, 1 out]
      }
      frame "select roi list" {
        n113 = Unbundle By Name(w323) -> ("Dimensions.Dim Z"=w325:i32)
        n114 = Variant To Data(error in=w300, type=i16 0, Variant=w301) -> (data=w299:i16, error out=w298:errorcluster)
        n115 = property on="ROIs Values Data" class="Arr (strict)"(error in=w298) -> (error out=w322:errorcluster, "Value"=w328:dbl[][])  [unwired: 1 in, 1 out]
        n116 = Less Or Equal To 0?(x=w325) -> (x <= 0?=w324:bool)
        n117 = property on="Z Slice" class="Slide (strict)"() -> ("Value"=w321:i16)  [unwired: 2 in, 2 out]
        n118 = Index Array(array=w328, index (row) #1=w299, index (col) #1=2 ("disabled index (col)"), index (row) #2=w299, index (col) #2=3 ("index (col)")) -> (element #1=w297:dbl, element #2=w296:dbl)
        n119 = case shown="False" w324 {
          tunnel: w320 -> [w336 w340]
          tunnel: w322 -> [w334 w339]
          tunnel: w323 -> [w335 w341]
          tunnel: [w334 w339] -> w318
          tunnel: [w332 w338] -> w319
          tunnel: w321 -> [w330 _]
          tunnel: w299 -> [w331 w337]
          frame False {
            n120 = call "extract roi 3d.vi"("ROI selected"=w331, "ROIs Array In"=w336, "Data Form"=w335) -> ("Table ROI 3D"=w333:i32[][][])  [unwired: 8 in]
            n121 = Index Array(array=w333, index (dim 0)=w330) -> (element=w332:i32[][])  [unwired: 2 in]
          }
          frame True {
            n122 = call "extract roi 2d.vi"("ROI selected"=w337, "ROIs Array In"=w340, "Data Form"=w341) -> ("Table ROI 2D"=w338:i32[][])  [unwired: 8 in]
          }
        }
        n123 = call "ROI Min Max.vi"("ROI 2"=w296, "ROI 1"=w297) -> ("ROI Max"=w294:dbl, "ROI Min"=w295:dbl)  [unwired: 8 in]
        n124 = property on="Intensity Graph" class="IntGraph (strict)"(error in=w318, "Value"=w319) -> (error out=w306:errorcluster)  [unwired: 1 in, 1 out]
        n125 = property on="Sum Spectrum" class="XYGraph (strict)"(error in=w306) -> (error out=w307:errorcluster, "Value"=w305:cluster{"Ramp Pattern":dbl[], "Array":i32[]}[], "CrsrList"=w303:T9)  [unwired: 1 in, 1 out]
        n126 = Index Array(array=w303, index #1=0 ("index"), index #2=1 ("index")) -> (element #1=w315:T10, element #2=w314:T10)
        n127 = Bundle By Name(cluster=w314, "Position.X"=w294) -> (w312:T10)
        n128 = Bundle By Name(cluster=w315, "Position.X"=w295) -> (w313:T10)
        n129 = call "area ROI.vi"("error in"=w307, "ROI max"=w294, "ROI min"=w295, "Sum Spectrum"=w305) -> ("error out"=w304:errorcluster, "XY Graph"=w309:cluster{"Channel":dbl[], "Intensity":i32[]}[])  [unwired: 5 in, 1 out]
        n130 = Build Array(w313, w312) -> (w308:T11)
        n131 = property on="Sum Spectrum" class="XYGraph (strict)"(error in=w304, "CrsrList"=w308) -> (error out=w310:errorcluster)  [unwired: 1 in, 1 out]
        n132 = property on="Sum Spectrum" class="XYGraph (strict)"(error in=w310, "Value"=w309) -> (error out=w311:errorcluster)  [unwired: 1 in, 1 out]
      }
      frame "zslice" {
        n133 = Variant To Data(error in=w350, type=i16 0 ("Z Slice"), Variant=w349) -> (data=w346:i16, error out=w343:errorcluster)
        n134 = property on="ROIs List" class="Ring (strict)"(error in=w343) -> (error out=w342:errorcluster, "Value"=w344:i16)  [unwired: 1 in, 1 out]
        n135 = call "extract roi 3d.vi"("ROI selected"=w344, "ROIs Array In"=w351, "Data Form"=w352) -> ("Table ROI 3D"=w347:i32[][][])  [unwired: 8 in]
        n136 = Index Array(array=w347, index (dim 0)=w346) -> (element=w345:i32[][])  [unwired: 2 in]
        n137 = property on="Intensity Graph" class="IntGraph (strict)"("Value"=w345) -> ()  [unwired: 2 in, 2 out]
      }
      frame "export" {
        n138 = Unbundle By Name(w363) -> ("Dimensions.Dim Z"=w364:i32, "Folder XRF Files"=w354:path)
        n139 = Less Or Equal To 0?(x=w364) -> (x <= 0?=w360:bool)
        n140 = Build Path(base path=w354, name or relative path=path "tables") -> (appended path=w359:path)
        n141 = call <vilib>:"Check if File or Folder Exists.vi"("path"=w359) -> ("file or folder exists?"=w357:bool, "dup path"=w358:path)  [unwired: 8 in, 1 out]
        n142 = case shown="False" w357 {
          tunnel: w358 -> [w368 w369]
          tunnel: [w367 w369] -> w356
          frame False {
            n143 = Create Folder(path (use dialog)=w368) -> (created path=w367:path)  [unwired: 2 in, 2 out]
          }
          frame True {
          }
        }
        n144 = case shown="False" w360 {
          tunnel: w362 -> [w372 w375]
          tunnel: [w371 w374] -> w361
          tunnel: w356 -> [w370 w373]
          frame False {
            n145 = call "elab pictures 3d.vi"("error in"=w372, "path file in"=w370) -> ("error out"=w371:errorcluster)  [unwired: 9 in]
          }
          frame True {
            n146 = call "elab pictures 2d.vi"("error in"=w375, "path file in"=w373) -> ("error out"=w374:errorcluster)  [unwired: 9 in]
          }
        }
      }
      frame "save" {
        n147 = Unbundle By Name(w382) -> ("Dimensions.Dim Z"=w392:i32, "Folder XRF Files"=w383:path)
        n148 = property on="Z Slice" class="Slide (strict)"() -> ("Value"=w377:i16)  [unwired: 2 in, 2 out]
        n149 = To Long Integer(number=w377) -> (32bit integer=w376:i32)
        n150 = Less Or Equal To 0?(x=w392) -> (x <= 0?=w389:bool)
        n151 = Build Path(base path=w383, name or relative path=path "tables") -> (appended path=w388:path)
        n152 = property on="ROIs List" class="Ring (strict)"() -> ("Strings []"=w380:string[], "Value"=w379:i16)  [unwired: 2 in, 2 out]
        n153 = call <vilib>:"Check if File or Folder Exists.vi"("path"=w388) -> ("file or folder exists?"=w386:bool, "dup path"=w387:path)  [unwired: 8 in, 1 out]
        n154 = Index Array(array=w380, index=w379) -> (element=w378:string)
        n155 = case shown="False" w386 {
          tunnel: w387 -> [w395 w396]
          tunnel: [w394 w396] -> w385
          frame False {
            n156 = Create Folder(path (use dialog)=w395) -> (created path=w394:path)  [unwired: 2 in, 2 out]
          }
          frame True {
          }
        }
        n157 = case shown="False" w389 {
          selector: w389 -> [w402 w415]
          tunnel: w391 -> [w403 w418]
          tunnel: [w405 w413] -> w390
          tunnel: w385 -> [w401 w417]
          tunnel: w382 -> [w410 w421]
          tunnel: w381 -> [w409 w420]
          tunnel: w379 -> [w408 w419]
          tunnel: w378 -> [w400 w416]
          tunnel: w376 -> [w407 _]
          frame False {
            n158 = call "extract roi 3d.vi"("ROI selected"=w408, "ROIs Array In"=w409, "Data Form"=w410) -> ("Table ROI 3D"=w406:i32[][][])  [unwired: 8 in]
            n159 = Index Array(array=w406, index (dim 0)=w407) -> (element=w397:i32[][])  [unwired: 2 in]
            n160 = Number To Decimal String(number=w407) -> (decimal integer string=w399:string)  [unwired: 1 in]
            n161 = call "name tables.vi"("2D?"=w402, "error in"=w403, "Z Slice"=w399, "ROI"=w400, "path folder in"=w401) -> ("error out"=w404:errorcluster, "path file out"=w398:path)  [unwired: 5 in]
            n162 = call-poly <vilib>:"Write Delimited Spreadsheet.vi"("file path (dialog if empty)"=w398, "2D data"=w397, "error in (no error)"=w404) -> ("error out"=w405:errorcluster)  [unwired: 11 in, 1 out]
          }
          frame True {
            n163 = call "extract roi 2d.vi"("ROI selected"=w419, "ROIs Array In"=w420, "Data Form"=w421) -> ("Table ROI 2D"=w412:i32[][])  [unwired: 8 in]
            n164 = call "name tables.vi"("2D?"=w415, "error in"=w418, "ROI"=w416, "path folder in"=w417) -> ("error out"=w414:errorcluster, "path file out"=w411:path)  [unwired: 6 in]
            n165 = call-poly <vilib>:"Write Delimited Spreadsheet.vi"("file path (dialog if empty)"=w411, "2D data"=w412, "error in (no error)"=w414) -> ("error out"=w413:errorcluster)  [unwired: 11 in, 1 out]
          }
        }
      }
      frame "saveall" {
        # "Va controllato con un 3D: quanti Z ci sono?"
        n166 = property on="Z Slice" class="Slide (strict)"() -> ("Scale.Maximum"=w425:dbl)  [unwired: 2 in, 2 out]
        n167 = Unbundle By Name(w427) -> ("Dimensions.Dim Z"=w437:i32, "Folder XRF Files"=w428:path)
        n168 = To Long Integer(number=w425) -> (32bit integer=w424:i32)
        n169 = Less Or Equal To 0?(x=w437) -> (x <= 0?=w434:bool)
        n170 = property on="ROIs List" class="Ring (strict)"() -> ("Strings []"=w423:string[])  [unwired: 2 in, 2 out]
        n171 = Build Path(base path=w428, name or relative path=path "tables") -> (appended path=w433:path)
        n172 = Decrement(x=w424) -> (x-1=w422:i32)
        n173 = call <vilib>:"Check if File or Folder Exists.vi"("path"=w433) -> ("file or folder exists?"=w431:bool, "dup path"=w432:path)  [unwired: 8 in, 1 out]
        n174 = case shown="False" w431 {
          tunnel: w432 -> [w483 w484]
          tunnel: [w482 w484] -> w430
          frame False {
            n175 = Create Folder(path (use dialog)=w483) -> (created path=w482:path)  [unwired: 2 in, 2 out]
          }
          frame True {
          }
        }
        n176 = for {
          tunnel: w434 -> [w445]
          tunnel: w430 -> [w444]
          tunnel: w427 -> [w443]
          tunnel: w426 -> [w442]
          tunnel: w423 -> [w441] mode=indexing
          tunnel: w422 -> [w440]
          shift-right: [w446] -> w435
          shift-left: w436 -> [w447]
          i -> [w439]
          n177 = case shown="False" w445 {
            selector: w445 -> [w451 w475]
            tunnel: w447 -> [w452 w478]
            tunnel: [w453 w473] -> w446
            tunnel: w444 -> [w450 w477]
            tunnel: w443 -> [w456 w481]
            tunnel: w442 -> [w455 w480]
            tunnel: w439 -> [w454 w479]
            tunnel: w441 -> [w449 w476]
            tunnel: w440 -> [w448 _]
            frame False {
              n178 = for {
                N: w448 -> [_]
                tunnel: w456 -> [w470]
                tunnel: w455 -> [w469]
                tunnel: w454 -> [w468]
                tunnel: w451 -> [w463]
                tunnel: w450 -> [w462]
                tunnel: w449 -> [w461]
                shift-right: [w466] -> w453
                shift-left: w452 -> [w464]
                i -> [w457]
                n179 = call "extract roi 3d.vi"("ROI selected"=w468, "ROIs Array In"=w469, "Data Form"=w470) -> ("Table ROI 3D"=w467:i32[][][])  [unwired: 8 in]
                n180 = Index Array(array=w467, index (dim 0)=w457) -> (element=w458:i32[][])  [unwired: 2 in]
                n181 = Number To Decimal String(number=w457) -> (decimal integer string=w460:string)  [unwired: 1 in]
                n182 = call "name tables.vi"("2D?"=w463, "error in"=w464, "Z Slice"=w460, "ROI"=w461, "path folder in"=w462) -> ("error out"=w465:errorcluster, "path file out"=w459:path)  [unwired: 5 in]
                n183 = call-poly <vilib>:"Write Delimited Spreadsheet.vi"("file path (dialog if empty)"=w459, "2D data"=w458, "error in (no error)"=w465) -> ("error out"=w466:errorcluster)  [unwired: 11 in, 1 out]
              }
            }
            frame True {
              n184 = call "extract roi 2d.vi"("ROI selected"=w479, "ROIs Array In"=w480, "Data Form"=w481) -> ("Table ROI 2D"=w472:i32[][])  [unwired: 8 in]
              n185 = call "name tables.vi"("2D?"=w475, "error in"=w478, "ROI"=w476, "path folder in"=w477) -> ("error out"=w474:errorcluster, "path file out"=w471:path)  [unwired: 6 in]
              n186 = call-poly <vilib>:"Write Delimited Spreadsheet.vi"("file path (dialog if empty)"=w471, "2D data"=w472, "error in (no error)"=w474) -> ("error out"=w473:errorcluster)  [unwired: 11 in, 1 out]
            }
          }
        }
      }
      frame "crop" {
        n187 = Unbundle By Name(w494) -> ("Dimensions.Dim Z"=w496:i32)
        n188 = property on="ROIs List" class="Ring (strict)"() -> ("Value"=w492:i16)  [unwired: 2 in, 2 out]
        n189 = property on="Z Slice" class="Slide (strict)"() -> ("Value"=w491:i16)  [unwired: 2 in, 2 out]
        n190 = Less Or Equal To 0?(x=w496) -> (x <= 0?=w495:bool)
        n191 = case shown="False" w495 {
          tunnel: w494 -> [w504 w509]
          tunnel: w493 -> [w503 w508]
          tunnel: w492 -> [w502 w507]
          tunnel: [w499 w506] -> w488
          tunnel: w491 -> [w501 _]
          tunnel: w490 -> [w498 w505]
          tunnel: [w498 w505] -> w489
          frame False {
            n192 = call "extract roi 3d.vi"("ROI selected"=w502, "ROIs Array In"=w503, "Data Form"=w504) -> ("Table ROI 3D"=w500:i32[][][])  [unwired: 8 in]
            n193 = Index Array(array=w500, index (dim 0)=w501) -> (element=w499:i32[][])  [unwired: 2 in]
          }
          frame True {
            n194 = call "extract roi 2d.vi"("ROI selected"=w507, "ROIs Array In"=w508, "Data Form"=w509) -> ("Table ROI 2D"=w506:i32[][])  [unwired: 8 in]
          }
        }
        n195 = property on="Intensity Graph" class="IntGraph (strict)"("Value"=w488) -> ()  [unwired: 2 in, 2 out]
        n196 = call "Crop Graph.vi"("error in"=w489, "Image In"=w488) -> ("error out"=w485:errorcluster, "Invert Roi"=→"Invert Roi XY":bool[], "Roi"=→"Roi XY":T1)  [unwired: 7 in]
      }
      frame "cropall" {
        n197 = Unbundle By Name(w523) -> ("Folder XRF Files"=w516:path, "Dimensions.Dim Z"=w525:i32)
        n198 = property on="ROIs List" class="Ring (strict)"(error in=w520) -> (error out=w518:errorcluster, "Strings []"=w519:string[])  [unwired: 1 in, 1 out]
        n199 = property on="Z Slice" class="Slide (strict)"() -> ("Scale.Maximum"=w512:dbl)  [unwired: 2 in, 2 out]
        n200 = property on="Roi XY" class="Clust (strict)"(error in=w518) -> (error out=w515:errorcluster, "Value"=w517:T1)  [unwired: 1 in, 1 out]
        n201 = To Long Integer(number=w512) -> (32bit integer=w511:i32)
        n202 = Decrement(x=w511) -> (x-1=w510:i32)
        n203 = Less Or Equal To 0?(x=w525) -> (x <= 0?=w524:bool)
        n204 = property on="Invert Roi XY" class="Arr (strict)"(error in=w515) -> (error out=w514:errorcluster, "Value"=w513:bool[])  [unwired: 1 in, 1 out]
        n205 = for {
          tunnel: w524 -> [w537]
          tunnel: w523 -> [w536]
          tunnel: w522 -> [w535]
          shift-right: [w534] -> w521
          shift-left: w514 -> [w533]
          tunnel: w519 -> [w530] mode=indexing
          tunnel: w517 -> [w531]
          tunnel: w516 -> [w529]
          tunnel: w513 -> [w528]
          tunnel: w510 -> [w527]
          i -> [w532]
          n206 = case shown="False" w537 {
            tunnel: w536 -> [w545 w574]
            tunnel: w535 -> [w544 w573]
            tunnel: w532 -> [w543 w572]
            tunnel: w533 -> [w542 w567]
            tunnel: [w541 w565] -> w534
            tunnel: w531 -> [_ w570]
            tunnel: w530 -> [w538 w561]
            tunnel: w529 -> [w540 w564]
            tunnel: w528 -> [_ w568]
            tunnel: w527 -> [w539 _]
            frame False {
              n207 = for {
                N: w539 -> [_]
                tunnel: w545 -> [w560]
                tunnel: w544 -> [w559]
                tunnel: w543 -> [w558]
                shift-right: [w548] -> w541
                shift-left: w542 -> [w547]
                tunnel: w540 -> [w552]
                tunnel: w538 -> [w550]
                i -> [w556]
                w546 = T5."Enabled" ("Disabled")
                n208 = property on="crop Z" class="Bool"("DisabledEnum"=w546) -> ()  [unwired: 2 in, 2 out]
                n209 = property on="Crop Z sl" class="Slide (strict)"("DisabledEnum"=w546) -> ()  [unwired: 2 in, 2 out]
                n210 = call "extract roi 3d.vi"("ROI selected"=w558, "ROIs Array In"=w559, "Data Form"=w560) -> ("Table ROI 3D"=w557:i32[][][])  [unwired: 8 in]
                n211 = Index Array(array=w557, index (dim 0)=w556) -> (element=w553:i32[][])  [unwired: 2 in]
                n212 = Number To Decimal String(number=w556) -> (decimal integer string=w551:string)  [unwired: 1 in]
                n213 = call "Crop Roi.vi"("Table Roi In"=w553) -> ("Table Roi Out"=w554:i32[][])  [unwired: 10 in]
                n214 = call "name tables.vi"("Z Slice"=w551, "ROI"=w550, "path folder in"=w552) -> ("path file out"=w549:path)  [unwired: 7 in, 1 out]
                n215 = call "Programmatically Invert Roi.vi"("Table Roi In"=w554) -> ("Table Roi Out"=w555:i32[][])  [unwired: 10 in]
                n216 = call-poly <vilib>:"Write Delimited Spreadsheet.vi"("file path (dialog if empty)"=w549, "2D data"=w555, "error in (no error)"=w547) -> ("error out"=w548:errorcluster)  [unwired: 11 in, 1 out]
              }
            }
            frame True {
              n217 = call "extract roi 2d.vi"("ROI selected"=w572, "ROIs Array In"=w573, "Data Form"=w574) -> ("Table ROI 2D"=w571:i32[][])  [unwired: 8 in]
              n218 = call "Crop Roi.vi"("Roi"=w570, "Table Roi In"=w571) -> ("Table Roi Out"=w569:i32[][])  [unwired: 9 in]
              n219 = call "Programmatically Invert Roi.vi"("Invert Roi"=w568, "Table Roi In"=w569) -> ("Table Roi Out"=w562:i32[][])  [unwired: 9 in]
              n220 = call "name tables.vi"("error in"=w567, "ROI"=w561, "path folder in"=w564) -> ("error out"=w566:errorcluster, "path file out"=w563:path)  [unwired: 7 in]
              n221 = call-poly <vilib>:"Write Delimited Spreadsheet.vi"("file path (dialog if empty)"=w563, "2D data"=w562, "error in (no error)"=w566) -> ("error out"=w565:errorcluster)  [unwired: 11 in, 1 out]
            }
          }
        }
      }
      frame "cropz" {
        n222 = Unbundle By Name(w577) -> ("Folder XRF Files"=w576:path)
        n223 = Variant To Data(error in=w583, type=cluster{"sl1":i32, "sl2":i32} {"sl1"=0, "sl2"=3} ("Crop Z"), Variant=w581) -> (data=w579:cluster{"sl1":i32, "sl2":i32}, error out=w580:errorcluster)
        n224 = call "delete z slices tabs.vi"("error in"=w580, "Crop Z"=w579, "File Table Folder"=w576) -> ("error out"=w575:errorcluster)  [unwired: 8 in]
      }
    }
  }
  n225 = while {
    shift-right: [w593] -> _
    shift-left: w5 -> [w594]
    shift-right: [w588] -> w8
    shift-left: w7 -> [w595]
    shift-right: [w587] -> _
    shift-left: _ -> [w586]
    tunnel: w2 -> [w585]
    stop <- w590 stop-if-true
    n226 = call "Dequeue Message.vi"("error in (no error)"=w595, "Message Queue"=w594) -> ("error out"=w592:errorcluster, "Message Data"=w589:variant, "Message"=w591:string, "dup Message Queue"=w593:refnum<queue>)  [unwired: 5 in, 1 out]
    n227 = case shown="\"select\"" w591 {
      tunnel: w592 -> [w597 w601 w607 w619 w631]
      tunnel: [FALSE FALSE TRUE FALSE FALSE] -> w590
      tunnel: w589 -> [_ _ _ w618 w630]
      tunnel: [w597 w600 w606 w610 w624] -> w588
      tunnel: [w596 w599 refnum<data-value> refnum ("data value reference out") w612 w628] -> w587
      tunnel: w586 -> [w596 _ w605 w614 w628]
      tunnel: w585 -> [_ _ _ _ w625]
      frame Default {
      }
      frame "initialize" {
        n228 = New Data Value Reference(data value=i32[][] [] ("Data Loaded"), error in=w601) -> (data value reference=w599:refnum<data-value>, error out=w600:errorcluster)
      }
      frame "stop" {
        n229 = Delete Data Value Reference(data value reference=w605, error in=w607) -> (error out=w606:errorcluster)  [unwired: 1 out]
      }
      frame "load data" {
        n230 = Variant To Data(error in=w619, type=T4 {"Dimensions"={"Dim X"=0, "Dim Y"=0, "Dim Z"=0}, "Folder XRF Files"=path "", "Dynamic Load"=FALSE, "Data From Vitruvio?"=TRUE} ("Data Form"), Variant=w618) -> (data=w615:T4, error out=w616:errorcluster)
        n231 = call "read maps.vi"("error in"=w616, "Data Form"=w615, "data value reference In"=w614) -> ("error out"=w611:errorcluster, "All Spectra"=→"Sum Spectrum":cluster{"Ramp Pattern":dbl[], "Array":i32[]}[], "data value reference out"=w612:refnum<data-value>)  [unwired: 6 in]
        n232 = property on="load data" class="Bool (strict)"(error in=w611, "Value"=FALSE ("load data")) -> (error out=w610:errorcluster)  [unwired: 1 in, 1 out]
      }
      frame "select" {
        n233 = Variant To Data(error in=w631, type=i32[][] [] ("ROIs Min Max"), Variant=w630) -> (data=w627:i32[][], error out=w626:errorcluster)
        n234 = call "somma roi.vi"("ROIs Min Max"=w627, "Data loaded reference In"=w628) -> ("ROIs Array Out"=w622:i32[][])  [unwired: 9 in]
        n235 = To Variant(anything=w622) -> (Variant=w621:variant)
        n236 = call "Enqueue Message (Single).vi"("error in (no error)"=w626, "Message Data"=w621, "Message"="roi table", "Message Queue"=w625) -> ("error out"=w624:errorcluster)  [unwired: 6 in, 1 out]
      }
    }
  }
  n237 = while {
    tunnel: w7 -> [w635]
    tunnel: w11 -> [w636]
    shift-right: [w633] -> _
    shift-left: TRUE -> [w634]
    stop <- w637 stop-if-true
    n238 = event shown="[22] \"crop Z\": Value Change" {
      selector: _ -> [_ _ _ _ _ _ _ _ _ _ _ _ _ _ _ _ _ _ _ _ _ _ _]
      dyn-events: _ -> [_ _ _ _ _ _ _ _ _ _ _ _ _ _ _ _ _ _ _ _ _ _ _]
      timeout: _ -> [_ _ _ _ _ _ _ _ _ _ _ _ _ _ _ _ _ _ _ _ _ _ _]
      tunnel: [FALSE w648 FALSE FALSE FALSE FALSE FALSE FALSE FALSE FALSE FALSE FALSE FALSE FALSE FALSE FALSE FALSE FALSE FALSE FALSE FALSE FALSE FALSE] -> w637
      tunnel: w636 -> [_ w649 w655 w671 _ w682 w696 _ _ w716 w739 w754 w767 _ w780 w789 w797 w800 w805 w810 w815 w820 w827]
      tunnel: w635 -> [_ w643 w654 w668 _ w684 w692 _ _ w713 w738 w755 w764 w772 w781 w787 w795 w801 w806 w811 w816 w821 w828]
      tunnel: w634 -> [w638 w640 w653 w670 _ w686 w698 w699 w706 w708 w740 w757 w769 w774 w783 w784 w792 _ _ _ _ _ _]
      tunnel: [w638 w640 w653 w670 w675 w686 w698 w699 w706 w708 w740 w757 w769 w774 w783 w784 w792 _ _ _ _ _ _] -> w633
      event Timeout {
        n239 = event-data() -> ()  [unwired: 1 in, 3 out]
      }
      event "Stop": Value Change {
        w644 = "stop" ("name")
        w648 = TRUE
        n240 = event-data() -> ()  [unwired: 1 in, 6 out]
        n241 = Unbundle By Name(w649) -> ("Main"=w645:refnum<queue>, "Data"=w646:refnum<queue>, "Support"=w647:refnum<queue>)
        n242 = call "Enqueue Message (Single).vi"("Priority Message? (F)"=w648, "error in (no error)"=w643, "Message"=w644, "Message Queue"=w647) -> ("error out"=w642:errorcluster)  [unwired: 6 in, 1 out]
        n243 = call "Enqueue Message (Single).vi"("Priority Message? (F)"=w648, "error in (no error)"=w642, "Message"=w644, "Message Queue"=w646) -> ("error out"=w641:errorcluster)  [unwired: 6 in, 1 out]
        n244 = call "Enqueue Message (Single).vi"("Priority Message? (F)"=w648, "error in (no error)"=w641, "Message"=w644, "Message Queue"=w645) -> ()  [unwired: 6 in, 2 out]
      }
      event "reset": Value Change {
        n245 = event-data() -> ()  [unwired: 1 in, 6 out]
        n246 = Two Button Dialog(message="Are you sure you want to reset?") -> (T button?=w651:bool)  [unwired: 2 in]
        n247 = case shown="True" w651 {
          tunnel: w655 -> [_ w664]
          tunnel: w654 -> [_ w659]
          frame False {
          }
          frame True {
            w656 = TRUE
            w660 = "initialize" ("name")
            n248 = Unbundle By Name(w664) -> ("Main"=w661:refnum<queue>, "Data"=w662:refnum<queue>, "Support"=w663:refnum<queue>)
            n249 = call "Enqueue Message (Single).vi"("Priority Message? (F)"=w656, "error in (no error)"=w659, "Message"=w660, "Message Queue"=w663) -> ("error out"=w658:errorcluster)  [unwired: 6 in, 1 out]
            n250 = call "Enqueue Message (Single).vi"("Priority Message? (F)"=w656, "error in (no error)"=w658, "Message"=w660, "Message Queue"=w662) -> ("error out"=w657:errorcluster)  [unwired: 6 in, 1 out]
            n251 = call "Enqueue Message (Single).vi"("Priority Message? (F)"=w656, "error in (no error)"=w657, "Message"=w660, "Message Queue"=w661) -> ()  [unwired: 6 in, 2 out]
          }
        }
      }
      event "reset ROI": Value Change {
        w665 = "reset roi" ("Message")
        n252 = event-data() -> ()  [unwired: 1 in, 6 out]
        n253 = Unbundle By Name(w671) -> ("Main"=w666:refnum<queue>, "Data"=w673:refnum<queue>, "Support"=w672:refnum<queue>)
        n254 = Select(t=w673, s=w670, f=w672) -> (s? t:f=w669:refnum<queue>)
        n255 = call "Enqueue Message (Single).vi"("error in (no error)"=w668, "Message"=w665, "Message Queue"=w669) -> ("error out"=w667:errorcluster)  [unwired: 7 in, 1 out]
        n256 = call "Enqueue Message (Single).vi"("error in (no error)"=w667, "Message"=w665, "Message Queue"=w666) -> ()  [unwired: 7 in, 2 out]
      }
      event Value Change {
        n257 = event-data() -> ()  [unwired: 1 in, 6 out]
        n258 = Unbundle By Name("Data Form") -> ("Dimensions.Dim Z"=w676:i32)
        n259 = Less Or Equal To 0?(x=w676) -> (x <= 0?=w675:bool)
        n260 = case shown="False" w675 {
          tunnel: w676 -> [w679 _]
          frame False {
            n261 = property on="Z Slice" class="Slide (strict)"("DisabledEnum"=T5."Enabled" ("Disabled"), "Scale.Maximum"=w679) -> ()  [unwired: 2 in, 2 out]
          }
          frame True {
          }
        }
      }
      event "manipulate files": Value Change {
        n262 = event-data() -> ()  [unwired: 1 in, 6 out]
        n263 = Unbundle By Name(w682) -> ("Main"=w681:refnum<queue>)
        n264 = call "Enqueue Message (Single).vi"("error in (no error)"=w684, "Message"="manipulate", "Message Queue"=w681) -> ()  [unwired: 7 in, 2 out]
      }
      event "load data": Value Change {
        w688 = "load data" ("Message")
        n265 = event-data() -> ()  [unwired: 1 in, 6 out]
        n266 = Unbundle By Name(w696) -> ("Main"=w689:refnum<queue>, "Data"=w695:refnum<queue>, "Support"=w694:refnum<queue>)
        n267 = property on="Data Form" class="Clust (strict)"() -> ("Value"=w691:T4)  [unwired: 2 in, 2 out]
        n268 = Select(t=w695, s=w698, f=w694) -> (s? t:f=w693:refnum<queue>)
        n269 = To Variant(anything=w691) -> (Variant=w687:variant)
        n270 = call "Enqueue Message (Single).vi"("error in (no error)"=w692, "Message Data"=w687, "Message"=w688, "Message Queue"=w693) -> ("error out"=w690:errorcluster)  [unwired: 6 in, 1 out]
        n271 = call "Enqueue Message (Single).vi"("error in (no error)"=w690, "Message Data"=w687, "Message"=w688, "Message Queue"=w689) -> ()  [unwired: 6 in, 2 out]
      }
      event "mapping": Value Change {
        n272 = event-data() -> ()  [unwired: 1 in, 6 out]
        n273 = property on="Sum Spectrum" class="XYGraph (strict)"("YScale.Mapping Mode"="mapping") -> ()  [unwired: 2 in, 2 out]
      }
      event "autoscale": Value Change {
        n274 = event-data() -> ()  [unwired: 1 in, 6 out]
        n275 = Select(t=0, s="autoscale", f=2) -> (s? t:f=w702:i32)
        n276 = property on="Sum Spectrum" class="XYGraph (strict)"("XScale.ScaleFit"=w702) -> ()  [unwired: 2 in, 2 out]
      }
      event "load calib": Value Change {
        n277 = event-data() -> ()  [unwired: 1 in, 6 out]
        n278 = property on="debug?" class="Bool (strict)"() -> ("Value"=w709:bool)  [unwired: 2 in, 2 out]
        n279 = case shown="False" w709 {
          tunnel: w713 -> [w723 w730]
          tunnel: [w719 w731] -> w712
          tunnel: [w718 w730] -> w710
          frame False {
            w726 = 1 ("disabled index (col)")
            n280 = call-poly <vilib>:"Read Delimited Spreadsheet.vi"("error in (no error)"=w723) -> ("all rows"=w729:string[][], "error out"=w718:errorcluster)  [unwired: 9 in, 4 out]
            n281 = Index Array(array=w729, index (row) #1=0 ("index (row)"), index (col) #1=w726, index (row) #2=1 ("index (row)"), index (col) #2=w726) -> (element #1=w727:string, element #2=w728:string)
            n282 = Fract/Exp String To Number(string=w727) -> (number=w720:dbl)  [unwired: 3 in, 1 out]
            n283 = Fract/Exp String To Number(string=w728) -> (number=w721:dbl)  [unwired: 3 in, 1 out]
            n284 = Bundle By Name(cluster=T2 {"Intercept"=0.0, "slope"=0.0} ("Param Calibrazione"), "Intercept"=w720, "slope"=w721) -> (w719:T2)
          }
          frame True {
            w731 = T2 {"Intercept"=-0.21934166219283543, "slope"=0.005683540223633324}  # Param Calibrazione
          }
        }
        n285 = To Variant(anything=w712) -> (Variant=w711:variant)
        n286 = Unbundle By Name(w716) -> ("Main"=w715:refnum<queue>)
        n287 = call "Enqueue Message (Single).vi"("error in (no error)"=w710, "Message Data"=w711, "Message"="load calib", "Message Queue"=w715) -> ()  [unwired: 6 in, 2 out]
      }
      event "load param": Value Change {
        n288 = event-data() -> ()  [unwired: 1 in, 6 out]
        n289 = case shown="False" "debug?" {
          tunnel: [w747 w751] -> w742
          tunnel: [w746 path "" ("new file path (Not A Path if cancelled)")] -> w741
          tunnel: w738 -> [w745 w751]
          frame False {
            n290 = flat-sequence {
              tunnel: w745 -> [w749]
              tunnel: [w749] -> w744
              frame #0 {
                n291 = One Button Dialog(message="Select \"NAME_calib.dat\"\nfile") -> ()  [unwired: 1 in, 1 out]
              }
            }
            n292 = call-poly <vilib>:"Read Delimited Spreadsheet.vi"("error in (no error)"=w744) -> ("new file path (Not A Path if cancelled)"=w746:path, "error out"=w747:errorcluster)  [unwired: 9 in, 4 out]
          }
          frame True {
          }
        }
        n293 = Unbundle By Name(w739) -> ("Main"=w737:refnum<queue>)
        n294 = call "reading external parameters.vi"("debug?"="debug?", "error in (no error)"=w742, "path _calib.dat"=w741) -> ("error out"=w732:errorcluster, "ROIs cluster"=w733:T3)  [unwired: 7 in]
        n295 = To Variant(anything=w733) -> (Variant=w735:variant)
        n296 = call "Enqueue Message (Single).vi"("error in (no error)"=w732, "Message Data"=w735, "Message"="load parameters", "Message Queue"=w737) -> ()  [unwired: 6 in, 2 out]
      }
      event "calibrate": Value Change {
        n297 = event-data() -> ()  [unwired: 1 in, 6 out]
        n298 = Unbundle By Name(w754) -> ("Main"=w753:refnum<queue>)
        n299 = call "Enqueue Message (Single).vi"("error in (no error)"=w755, "Message"="calibrate", "Message Queue"=w753) -> ()  [unwired: 7 in, 2 out]
      }
      event "Edit ROI": Value Change {
        n300 = event-data() -> ()  [unwired: 1 in, 6 out]
        n301 = Unbundle By Name(w767) -> ("Main"=w766:refnum<queue>)
        n302 = property on="data ROIs" class="Clust (strict)"() -> ("Value"=w758:T3)  [unwired: 2 in, 2 out]
        n303 = property on="Calibration" class="Clust (strict)"() -> ("Value"=w760:T2)  [unwired: 2 in, 2 out]
        n304 = property on="Sum Spectrum" class="XYGraph (strict)"() -> ("Value"=w759:cluster{"Ramp Pattern":dbl[], "Array":i32[]}[])  [unwired: 2 in, 2 out]
        n305 = call "editroi.vi"("error in"=w764, "Calibration"=w760, "data ROIs"=w758, "Sum Spectrum"=w759) -> ("error out"=w763:errorcluster, "data ROIs out"=w762:T3)  [unwired: 6 in]
        n306 = To Variant(anything=w762) -> (Variant=w761:variant)
        n307 = call "Enqueue Message (Single).vi"("error in (no error)"=w763, "Message Data"=w761, "Message"="edit", "Message Queue"=w766) -> ()  [unwired: 6 in, 2 out]
      }
      event "area ROI": Value Change {
        n308 = event-data() -> ("NewVal"=w771:bool)  [unwired: 1 in, 5 out]
        n309 = property on="Sum Spectrum" class="XYGraph (strict)"(error in=w772, "Active Plot"=u32 1, "Plot.Visible?"=w771, "Active Plot"=u32 0) -> ()  [unwired: 1 in, 2 out]
      }
      event "Z Slice": Value Change {
        n310 = event-data() -> ()  [unwired: 1 in, 6 out]
        n311 = Unbundle By Name(w780) -> ("Main"=w779:refnum<queue>)
        n312 = To Variant(anything="Z Slice") -> (Variant=w776:variant)
        n313 = call "Enqueue Message (Single).vi"("error in (no error)"=w781, "Message Data"=w776, "Message"="zslice", "Message Queue"=w779) -> ()  [unwired: 6 in, 2 out]
      }
      event "ROIs Values": Mouse Up {
        n314 = event-data() -> ()  [unwired: 1 in, 8 out]
        n315 = Unbundle By Name(w789) -> ("Main"=w788:refnum<queue>)
        n316 = call "Enqueue Message (Single).vi"("error in (no error)"=w787, "Message"="select roi", "Message Queue"=w788) -> ()  [unwired: 7 in, 2 out]
      }
      event "ROIs List": Value Change {
        n317 = event-data() -> ("NewVal"=w791:i16)  [unwired: 1 in, 5 out]
        n318 = Unbundle By Name(w797) -> ("Main"=w796:refnum<queue>)
        n319 = To Variant(anything=w791) -> (Variant=w790:variant)
        n320 = call "Enqueue Message (Single).vi"("error in (no error)"=w795, "Message Data"=w790, "Message"="select roi list", "Message Queue"=w796) -> ()  [unwired: 6 in, 2 out]
      }
      event "export": Value Change {
        n321 = event-data() -> ()  [unwired: 1 in, 6 out]
        n322 = Unbundle By Name(w800) -> ("Main"=w799:refnum<queue>)
        n323 = call "Enqueue Message (Single).vi"("error in (no error)"=w801, "Message"="export", "Message Queue"=w799) -> ()  [unwired: 7 in, 2 out]
      }
      event "save": Value Change {
        n324 = event-data() -> ()  [unwired: 1 in, 6 out]
        n325 = Unbundle By Name(w805) -> ("Main"=w804:refnum<queue>)
        n326 = call "Enqueue Message (Single).vi"("error in (no error)"=w806, "Message"="save", "Message Queue"=w804) -> ()  [unwired: 7 in, 2 out]
      }
      event "save all": Value Change {
        n327 = event-data() -> ()  [unwired: 1 in, 6 out]
        n328 = Unbundle By Name(w810) -> ("Main"=w809:refnum<queue>)
        n329 = call "Enqueue Message (Single).vi"("error in (no error)"=w811, "Message"="saveall", "Message Queue"=w809) -> ()  [unwired: 7 in, 2 out]
      }
      event "crop": Value Change {
        n330 = event-data() -> ()  [unwired: 1 in, 6 out]
        n331 = Unbundle By Name(w815) -> ("Main"=w814:refnum<queue>)
        n332 = call "Enqueue Message (Single).vi"("error in (no error)"=w816, "Message"="crop", "Message Queue"=w814) -> ()  [unwired: 7 in, 2 out]
      }
      event "crop all": Value Change {
        n333 = event-data() -> ()  [unwired: 1 in, 6 out]
        n334 = Unbundle By Name(w820) -> ("Main"=w819:refnum<queue>)
        n335 = call "Enqueue Message (Single).vi"("error in (no error)"=w821, "Message"="cropall", "Message Queue"=w819) -> ()  [unwired: 7 in, 2 out]
      }
      event "crop Z": Value Change {
        n336 = event-data() -> ()  [unwired: 1 in, 6 out]
        n337 = Unbundle By Name(w827) -> ("Main"=w826:refnum<queue>)
        n338 = To Variant(anything="Crop Z sl") -> (Variant=w823:variant)
        n339 = call "Enqueue Message (Single).vi"("error in (no error)"=w828, "Message Data"=w823, "Message"="cropz", "Message Queue"=w826) -> ()  [unwired: 6 in, 2 out]
      }
    }
  }
  n340 = disable-structure shown="Disabled" {
    frame Disabled {
      n341 = property on="ROIs List" class="Ring (strict)" props=["Value"]() -> ()  [unwired: 2 in, 3 out]
      n342 = property on="Invert Roi XY" class="Arr (strict)" props=["Value"]() -> ()  [unwired: 2 in, 3 out]
      n343 = property on="Intensity Graph" class="IntGraph (strict)" props=["Value"]() -> ()  [unwired: 3 in, 2 out]
      n344 = property on="ROIs List" class="Ring (strict)" props=["StringsAndValues[]"]() -> ()  [unwired: 3 in, 2 out]
      n345 = property on="Sum Spectrum" class="XYGraph (strict)"("Active Plot"=u32 1, "Plot.Visible?"=FALSE ("Plot.Visible")) -> ()  [unwired: 2 in, 2 out]
      n346 = Unbundle By Name() -> ("Dimensions.Dim Z"=w832:i32)  [unwired: 1 in]
      n347 = Unbundle By Name() -> ("Data"=w834:refnum<queue>, "Support"=w835:refnum<queue>)  [unwired: 1 in]
      n348 = property on="Z Slice" class="Slide (strict)" props=["Value"]() -> ()  [unwired: 2 in, 3 out]
      n349 = call "read maps.vi"() -> ()  [unwired: 9 in, 3 out]
      n350 = property on="Roi XY" class="Clust (strict)" props=["Value"]() -> ()  [unwired: 2 in, 3 out]
      n351 = property on="debug?" class="Bool (strict)" props=["Value"]() -> ()  [unwired: 2 in, 3 out]
      n352 = Less Or Equal To 0?(x=w832) -> (x <= 0?=w833:bool)
      n353 = Select(t=w834, f=w835) -> ()  [unwired: 1 in, 1 out]
      n354 = Select(s=w833) -> ()  [unwired: 2 in, 1 out]
      n355 = call "Enqueue Message (Single).vi"() -> ()  [unwired: 10 in, 2 out]
      n356 = property on="debug?" class="Bool (strict)" props=["Value"]() -> ()  [unwired: 3 in, 2 out]
      n357 = call "extract roi 2d.vi"() -> ()  [unwired: 11 in, 1 out]
      n358 = call "extract roi 3d.vi"() -> ()  [unwired: 11 in, 1 out]
    }
    frame Enabled {
    }
  }
  n359 = Merge Errors(w4, w8, w9) -> (→"error out":errorcluster)
